vi "test.vi"() -> ()   [LabVIEW 2017]
uses:
  <vilib>/imath/engines/lvmath/Functions/Error Handling/error.ctl
  <vilib>/imath/engines/lvmath2/RunTimeEngine/Managers/WorkSpace/UID Generator.vi
  <vilib>/imath/engines/lvmath2/RunTimeEngine/NonStaticBuiltInFunctions/Manual/NIMS_NS_load.vi
  <vilib>/imath/engines/lvmath2/RunTimeEngine/NonStaticBuiltInFunctions/Manual/NIMS_NS_plot.vi
  <vilib>/imath/engines/lvmath2/RunTimeEngine/NonStaticBuiltInFunctions/NIMS_NS_hold.vi
  <vilib>/imath/engines/lvmath2/RunTimeEngine/NonStaticBuiltInFunctions/Manual/NIMS_NS_xlabel.vi
  <vilib>/imath/engines/lvmath2/RunTimeEngine/NonStaticBuiltInFunctions/Manual/NIMS_NS_ylabel.vi
  <vilib>/imath/engines/lvmath2/RunTimeEngine/NonStaticBuiltInFunctions/Manual/NIMS_NS_title.vi
  <vilib>/imath/engines/lvmath2/RunTimeEngine/NonStaticBuiltInFunctions/NIMS_NS_grid.vi
  <vilib>/imath/engines/lvmath2/RunTimeEngine/NonStaticBuiltInFunctions/Manual/NIMS_NS_legend.vi
  <vilib>/imath/engines/lvmath2/RunTimeEngine/RunTimeSymbolToken/NIMS_RunTimeSymbolToken_ResolveSymbol.vi
  <instcachedir>/0/NIMS_RunTimeSymbolToken_ResolveSymbol_AC7761ED747449B086FD7FB12AB2CB90.lvgen/NIMS_RunTimeSymbolToken_ResolveSymbol_AC7761ED747449B086FD7FB12AB2CB90_003.vi
  <vilib>/imath/engines/lvmath2/RunTimeEngine/Managers/SymbolTable/Write Variable.vi
  <vilib>/imath/engines/lvmath2/RunTimeEngine/Managers/SymbolTable/Read Variable.vi
  <vilib>/imath/engines/lvmath2/RunTimeEngine/VariableToken/Read/NIMS_Get Elements - _($,_) - nonstatic.vi
  <vilib>/imath/engines/lvmath2/RunTimeEngine/RunTimeSymbolToken/NIMS_RunTimeSymbolToken_UserFunctionInvoke.vi
  <vilib>/imathl/engines/lvmath/Functions/Error Handling/Create Error.vi
  <vilib>/imath/engines/lvmath2/RunTimeEngine/ArithmeticOperatorToken/NIMS_NS_ArithmeticOperator_times.vi
  <vilib>/imath/engines/lvmath/Functions/Error Handling/MergeErrorsWrapper.vi
  <instcachedir>/0/NIMS_RunTimeSymbolToken_ResolveSymbol_AC7761ED747449B086FD7FB12AB2CB90.lvgen/NIMS_RunTimeSymbolToken_ResolveSymbol_AC7761ED747449B086FD7FB12AB2CB90_002.vi
  <instcachedir>/0/NIMS_RunTimeSymbolToken_ResolveSymbol_AC7761ED747449B086FD7FB12AB2CB90.lvgen/NIMS_RunTimeSymbolToken_ResolveSymbol_AC7761ED747449B086FD7FB12AB2CB90_000.vi
  <vilib>/imath/engines/lvmath2/RunTimeEngine/CommandStatement/NIMS_CommandStatement_MaskErr.vi
  <vilib>/imath/engines/lvmath2/RunTimeEngine/NodeEndStatement/MC_NodeEndStatement_Dispose.vi
  <vilib>/imath/engines/lvmath2/RunTimeEngine/ErrorHandling/NIMS_Finalize Error.vi
  <vilib>/imath/engines/lvmath2/RunTimeEngine/ArithmeticOperatorToken/NIMS_NS_ArithmeticOperator_plus.vi
  <vilib>/imath/engines/lvmath2/RunTimeEngine/ArithmeticOperatorToken/NIMS_NS_ArithmeticOperator_minus.vi
  <vilib>/imath/engines/lvmath2/RunTimeEngine/Managers/SymbolTable/NIMS_WorkSpace.lvlib
panel:
  in  "还原按钮":bool
  in  "电机工作频率":dbl
  in  "预紧力":dbl
  in  "转子光电总阻尼":dbl
  in  "轴向阻尼系数":dbl
  in  "转子等效半径":dbl
  in  "输入完成":bool
  in  "摩擦材料等效刚度":dbl
  in  "定转子间动摩擦系数":dbl
  in  "行波波数":dbl
  out "loading":T1 caption="Loading..." scale=0.0..100.0
  in  "摩擦转矩-转速":bool
  in  "启动特性":bool
  in  "完成":bool
  in  "完成":bool
  in  "完成":bool
  in  "矩角特性":bool
  in  "?":bool
  in  "?":bool
  in  "?":bool
  in  "定子形波振幅3":dbl
  in  "定子形波振幅2":dbl
  in  "定子形波振幅":dbl
  in  "启动特性":bool
  in  "完成":bool
  in  "?":bool
  in  "负载转矩4":dbl
  in  "完成":bool
  in  "完成":bool
  in  "完成":bool
  in  "矩角特性":bool
  in  "净输出转矩-转速关系":bool
  in  "?":bool
  in  "?":bool
  in  "?":bool
  in  "负载转矩3":dbl
  in  "负载转矩2":dbl
  in  "负载转矩1":dbl
  in  "完成":bool
  in  "完成":bool
  in  "完成":bool
  in  "启动特性":bool
  in  "矩角特性":bool
  in  "?":bool
  in  "?":bool
  in  "?":bool
  in  "转动惯量":dbl
  in  "转动惯量":dbl
  in  "转动惯量":dbl
  # "瞬态特性测试模块"
  # "负载转矩"
  # "电机参数"
  # "负载转动惯量"
  # "定子行波振幅"
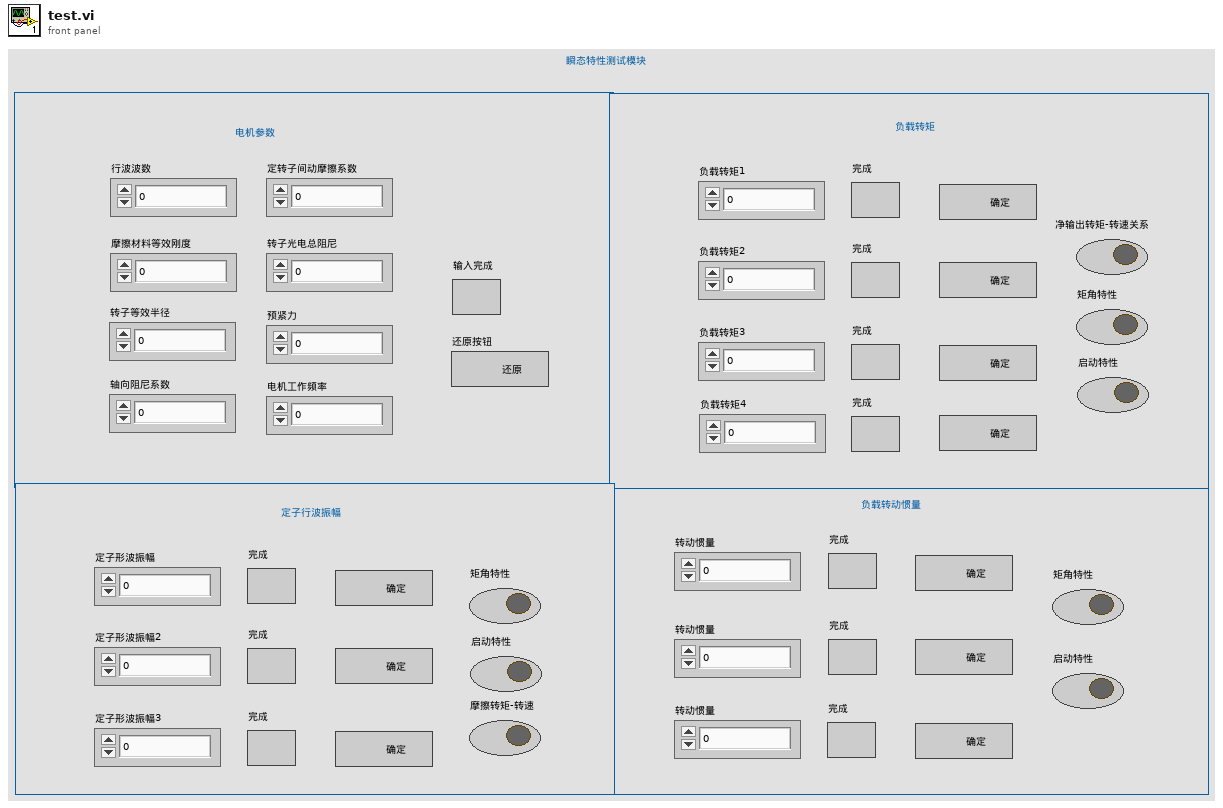
[diagram p1: front panel]
types:
  T1 = typedef "控件 1.ctl" = u8
  T2 = enum16{"open", "replace", "create", "open or create", "replace or create", "replace or create with confirmation"}
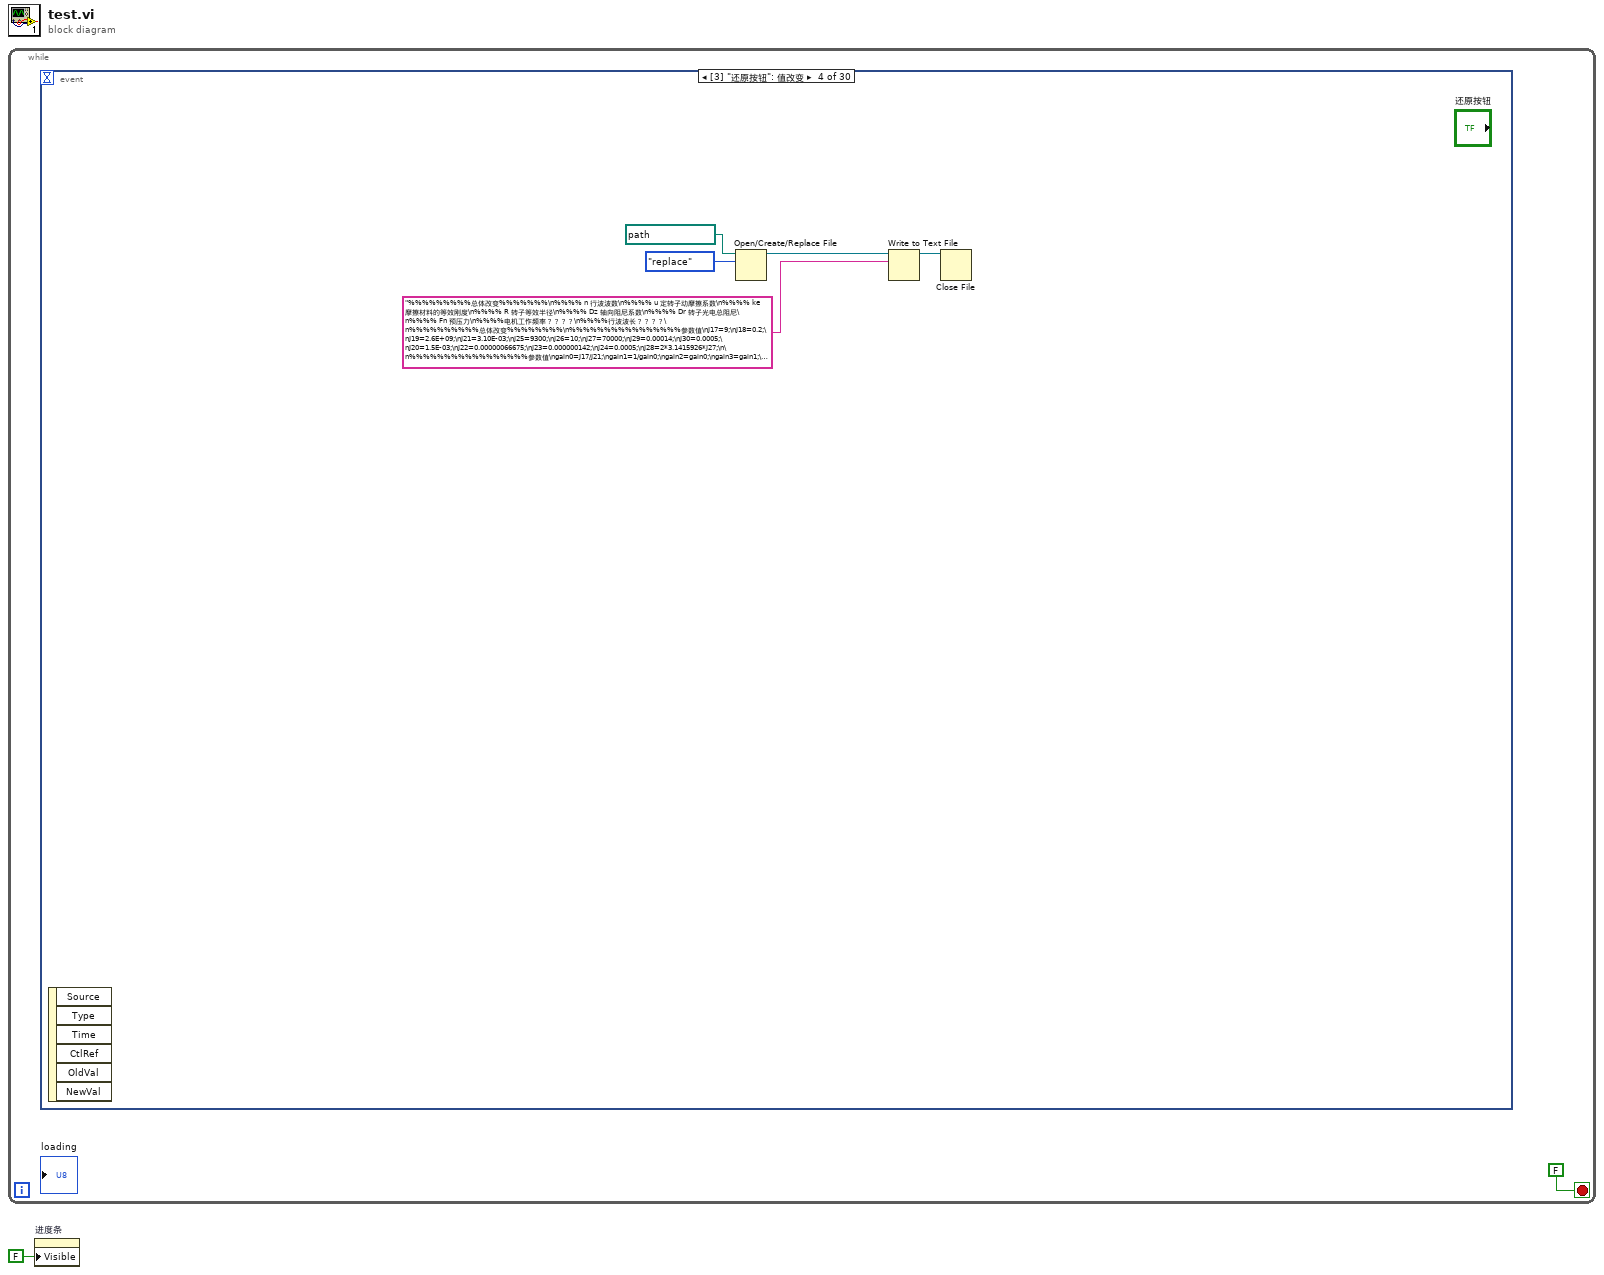
[diagram p0: block diagram]
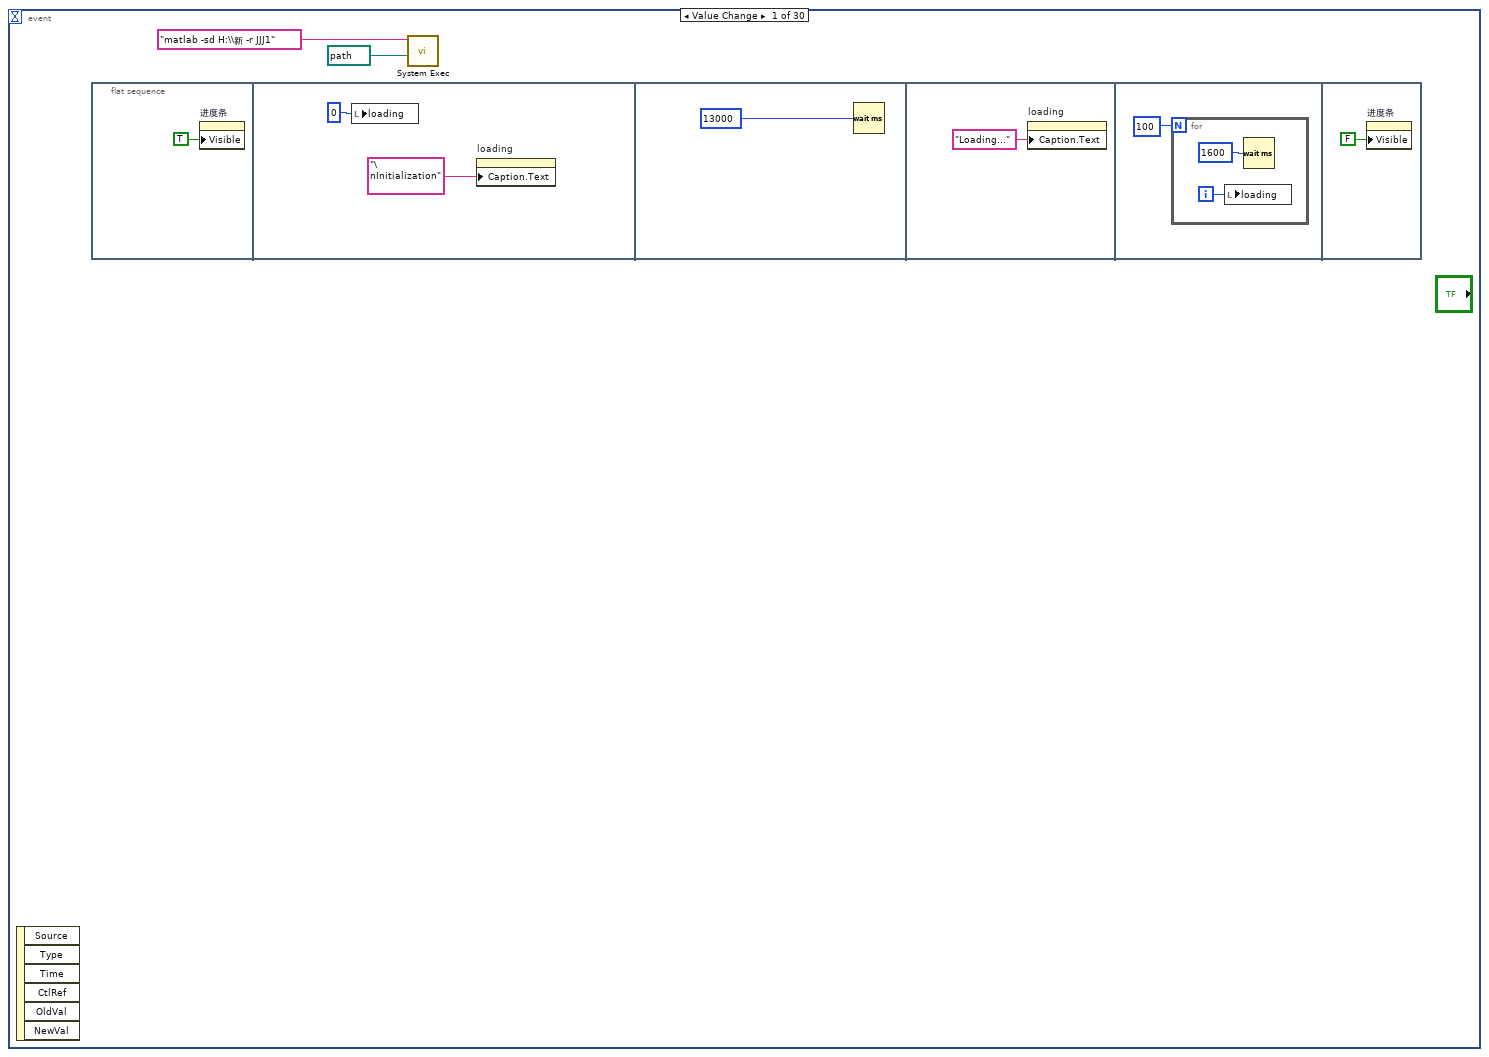
[diagram p2: hidden frame]
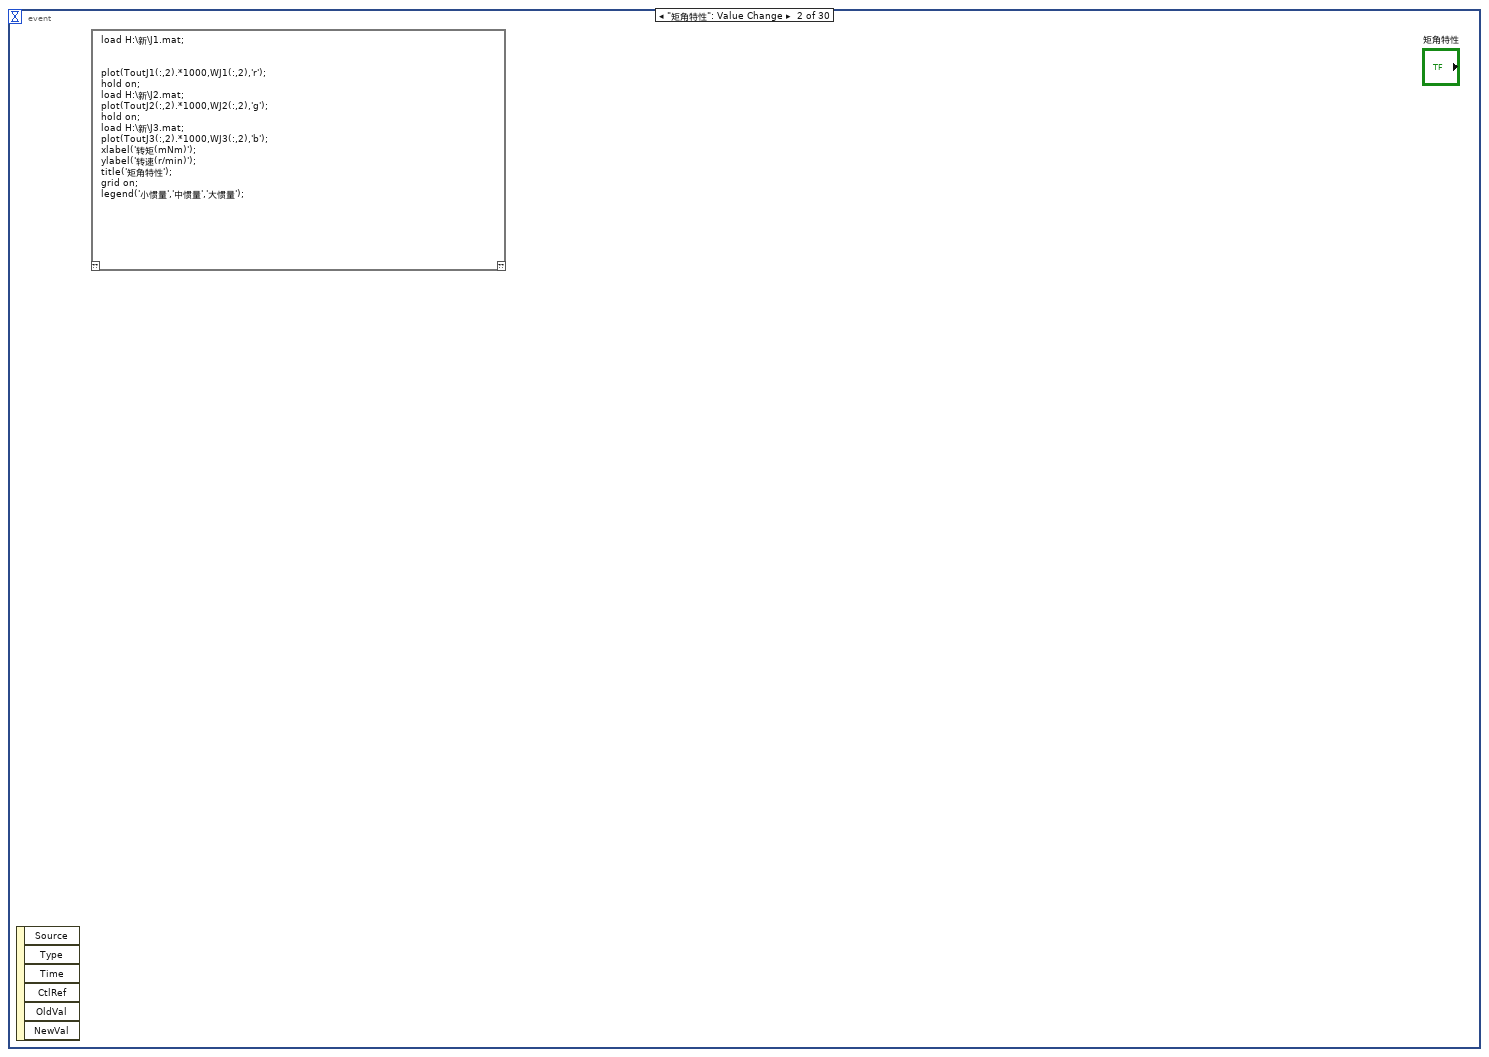
[diagram p3: hidden frame]
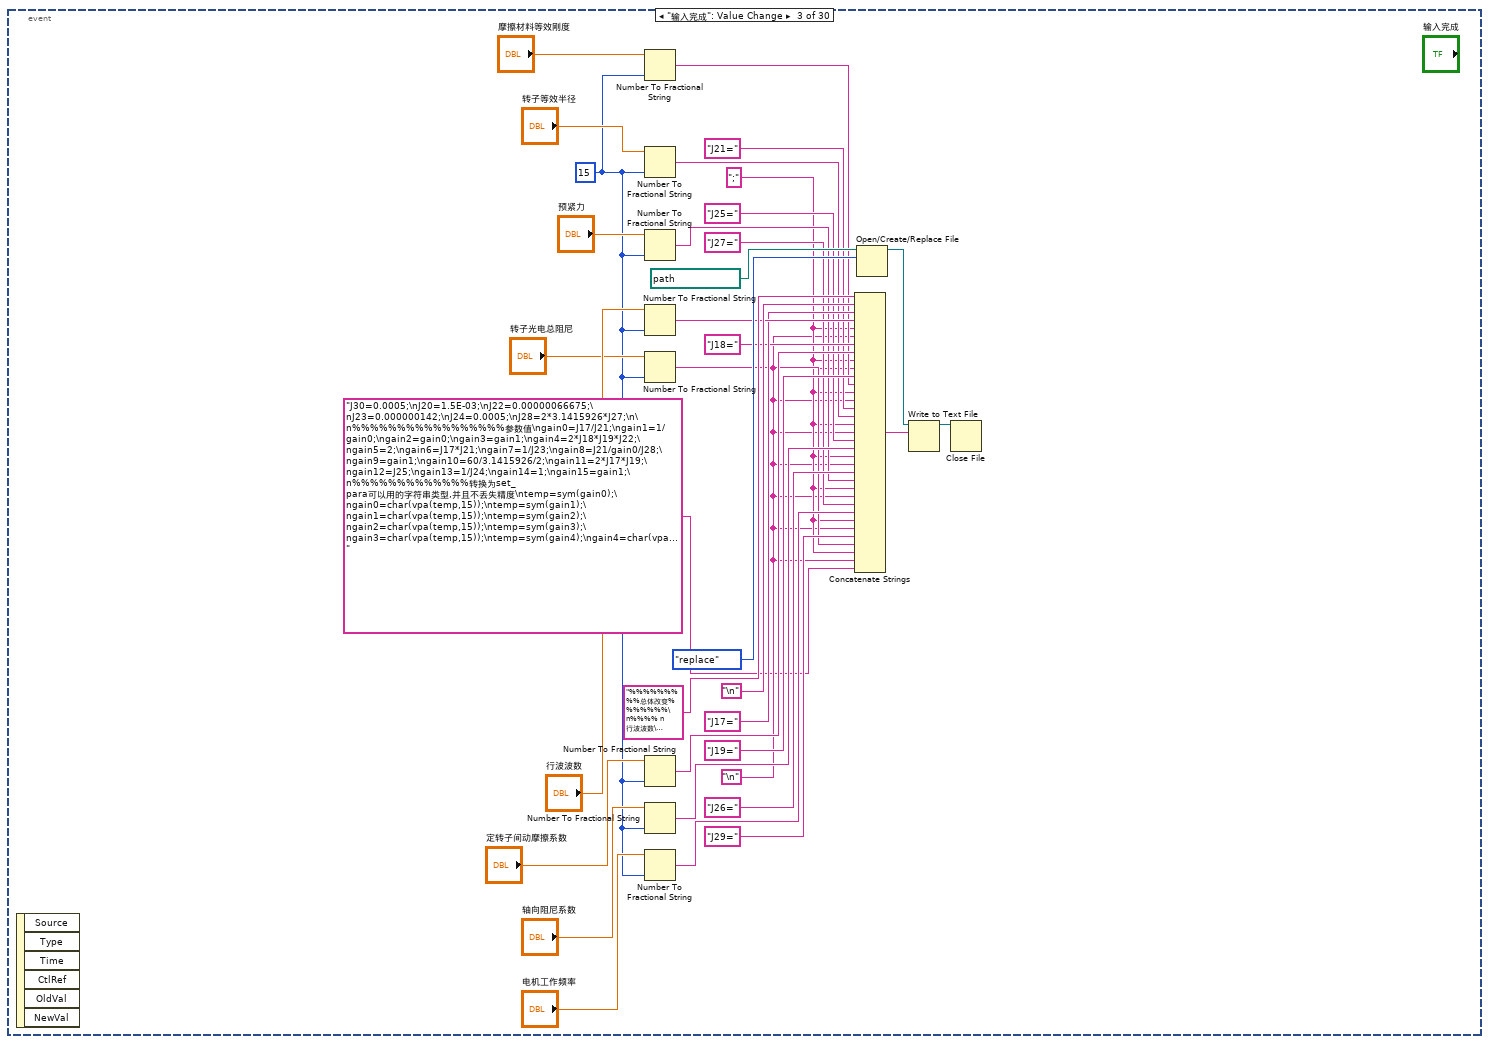
[diagram p4: hidden frame]
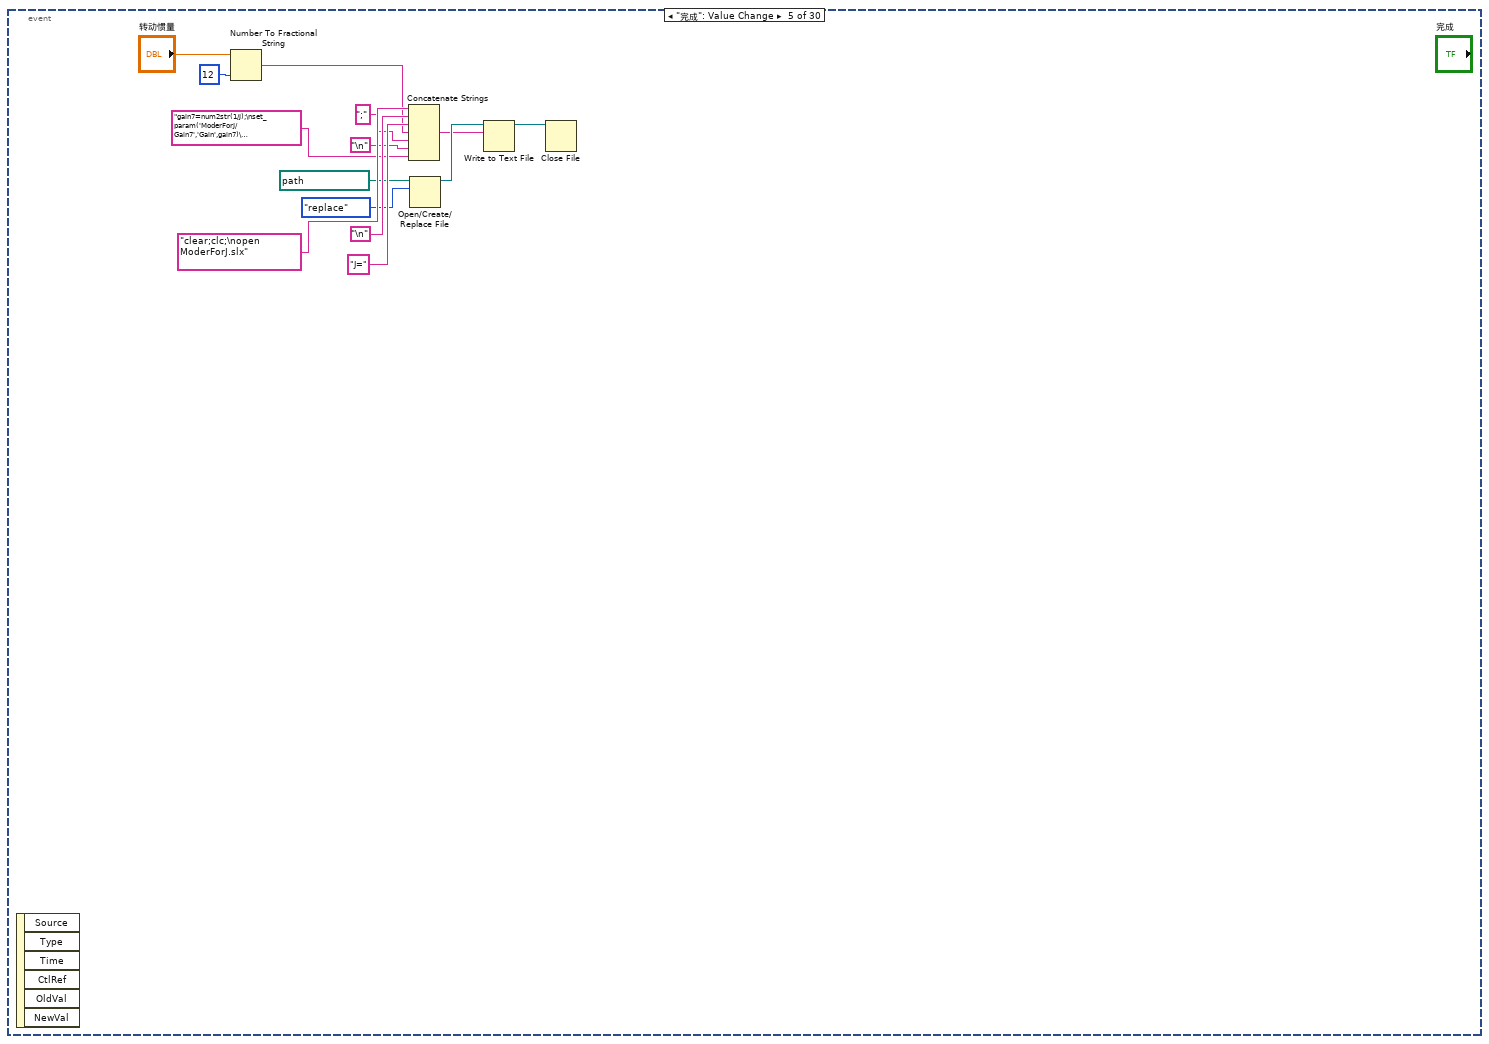
[diagram p5: hidden frame]
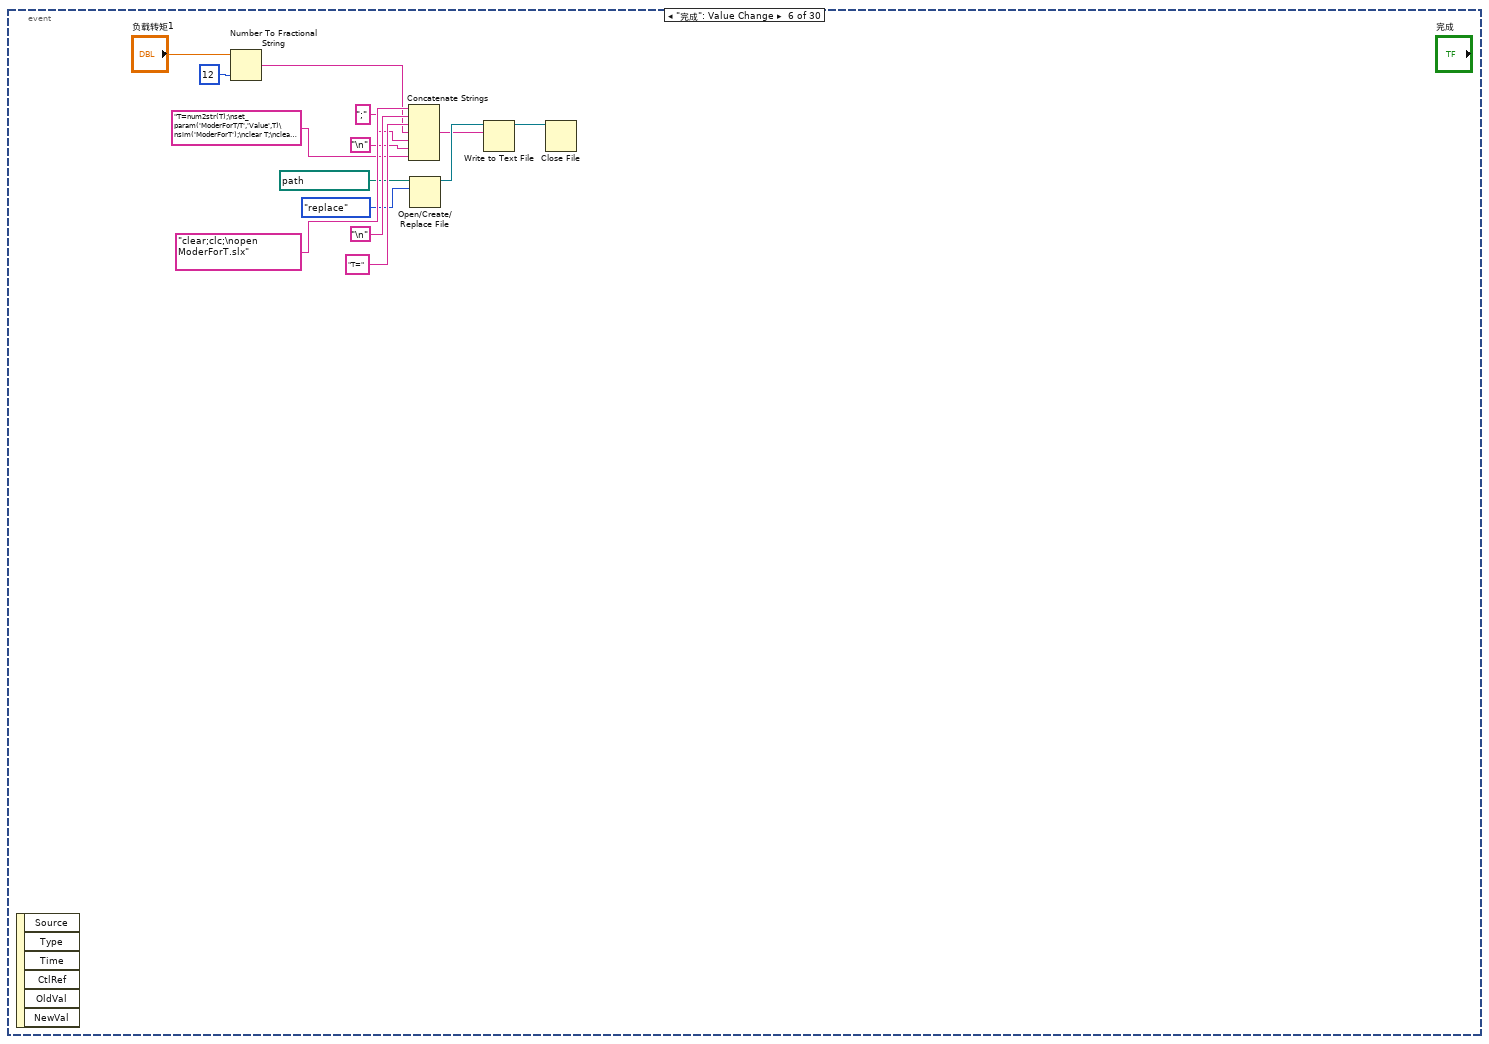
[diagram p6: hidden frame]
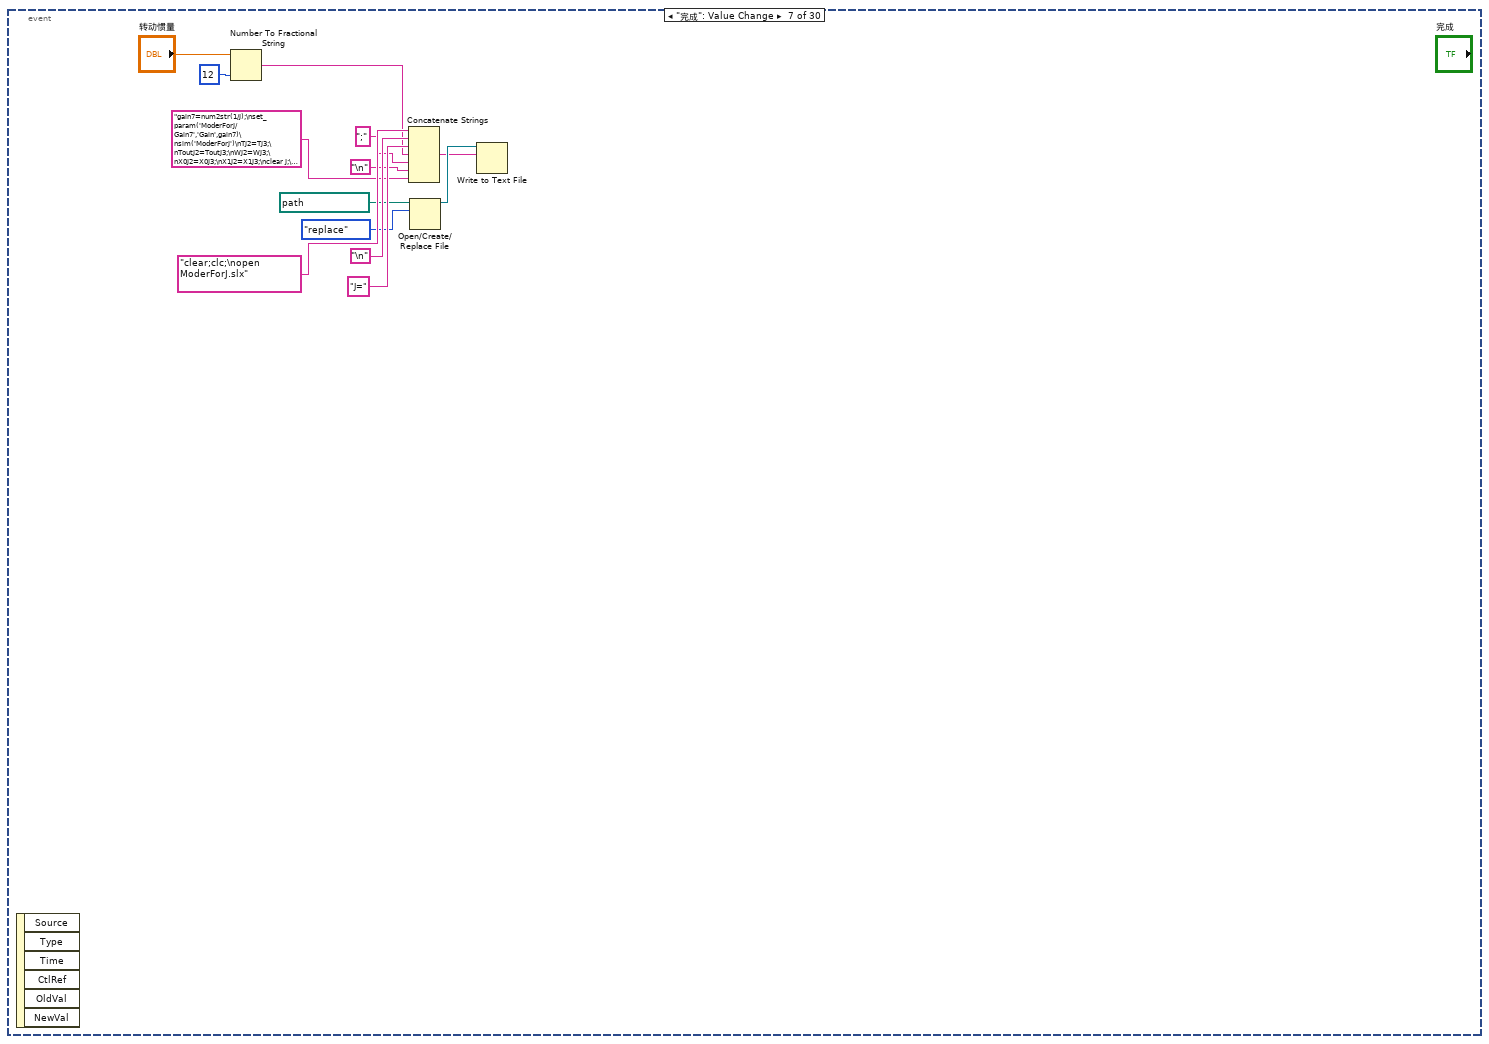
[diagram p7: hidden frame]
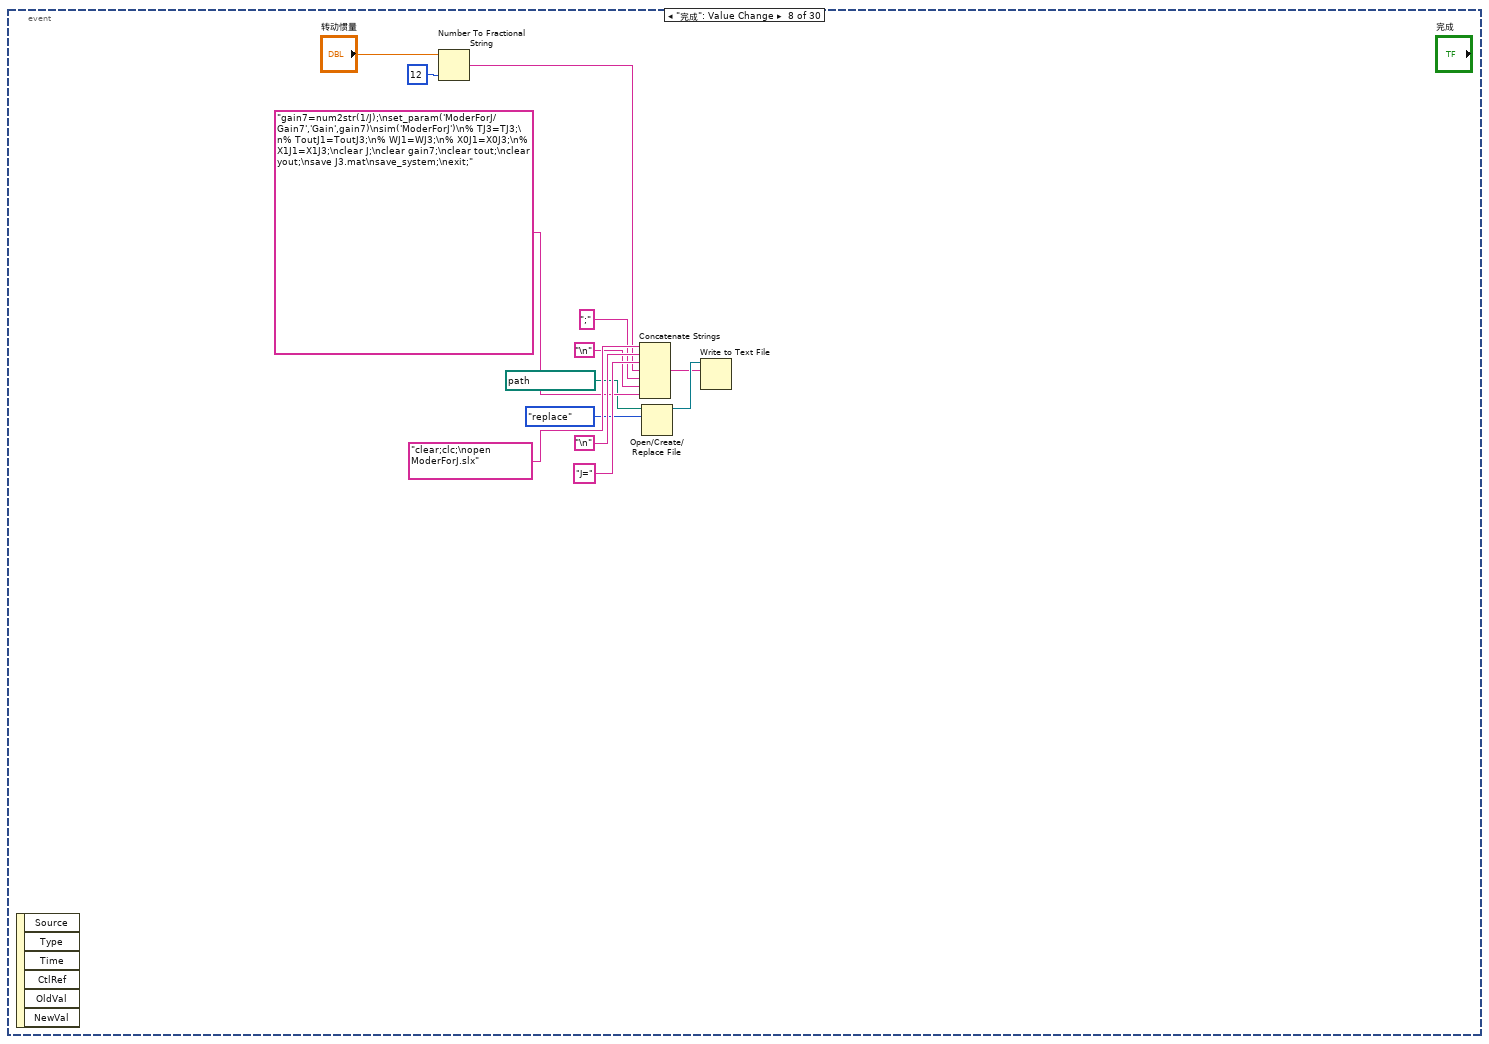
[diagram p8: hidden frame]
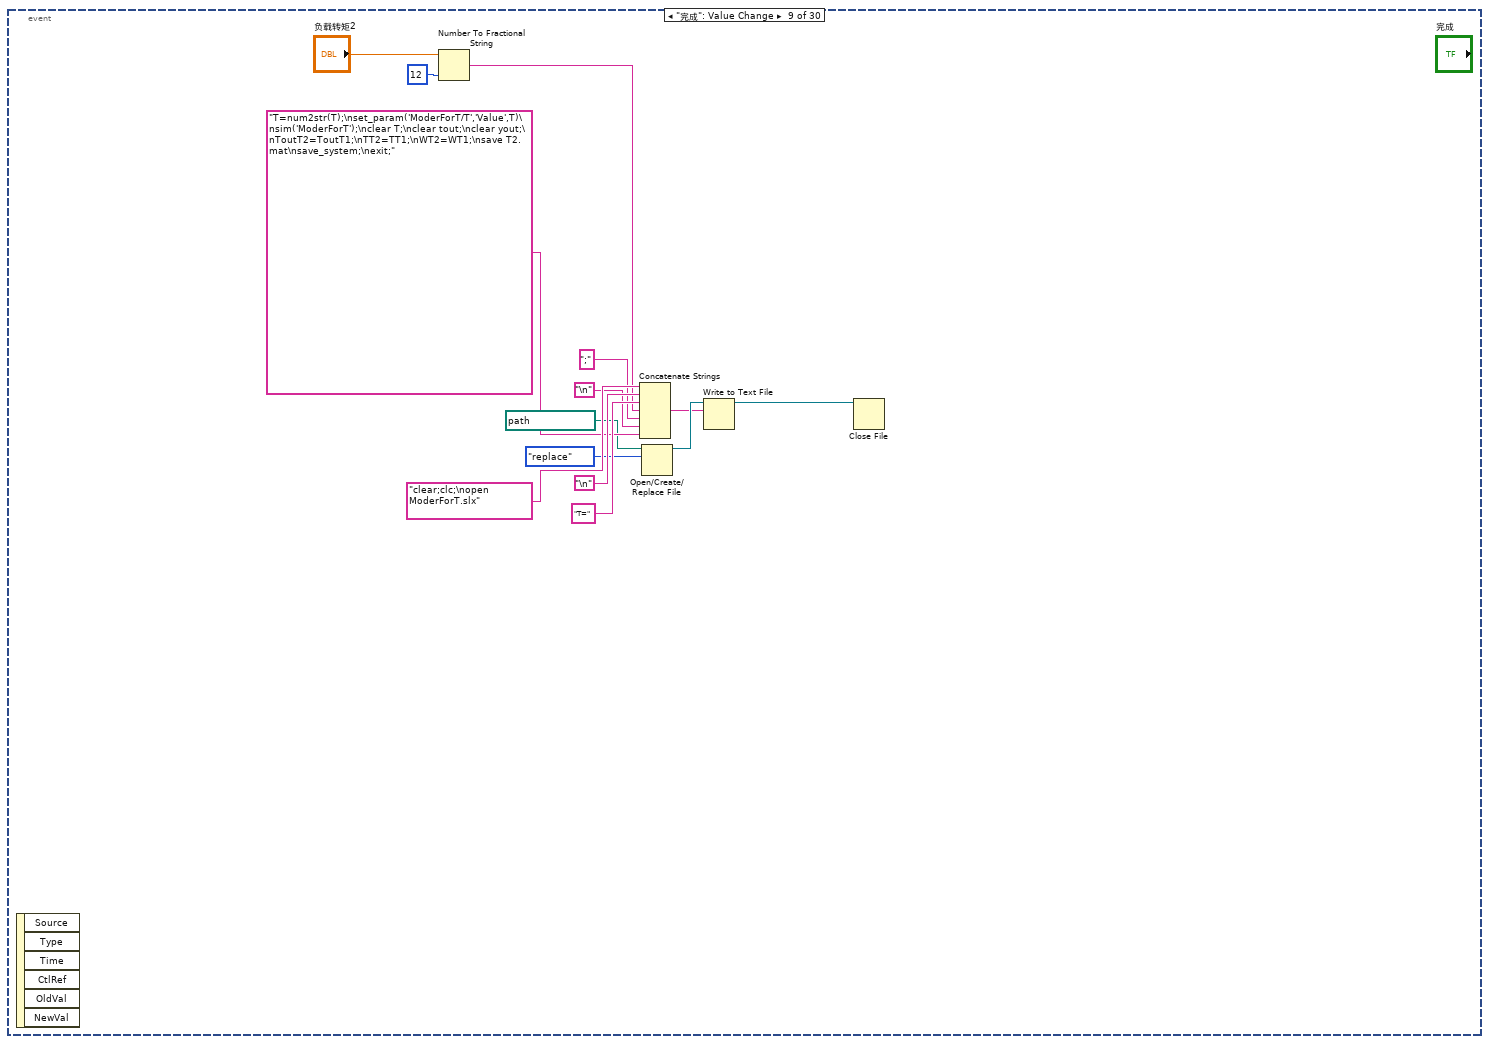
[diagram p9: hidden frame]
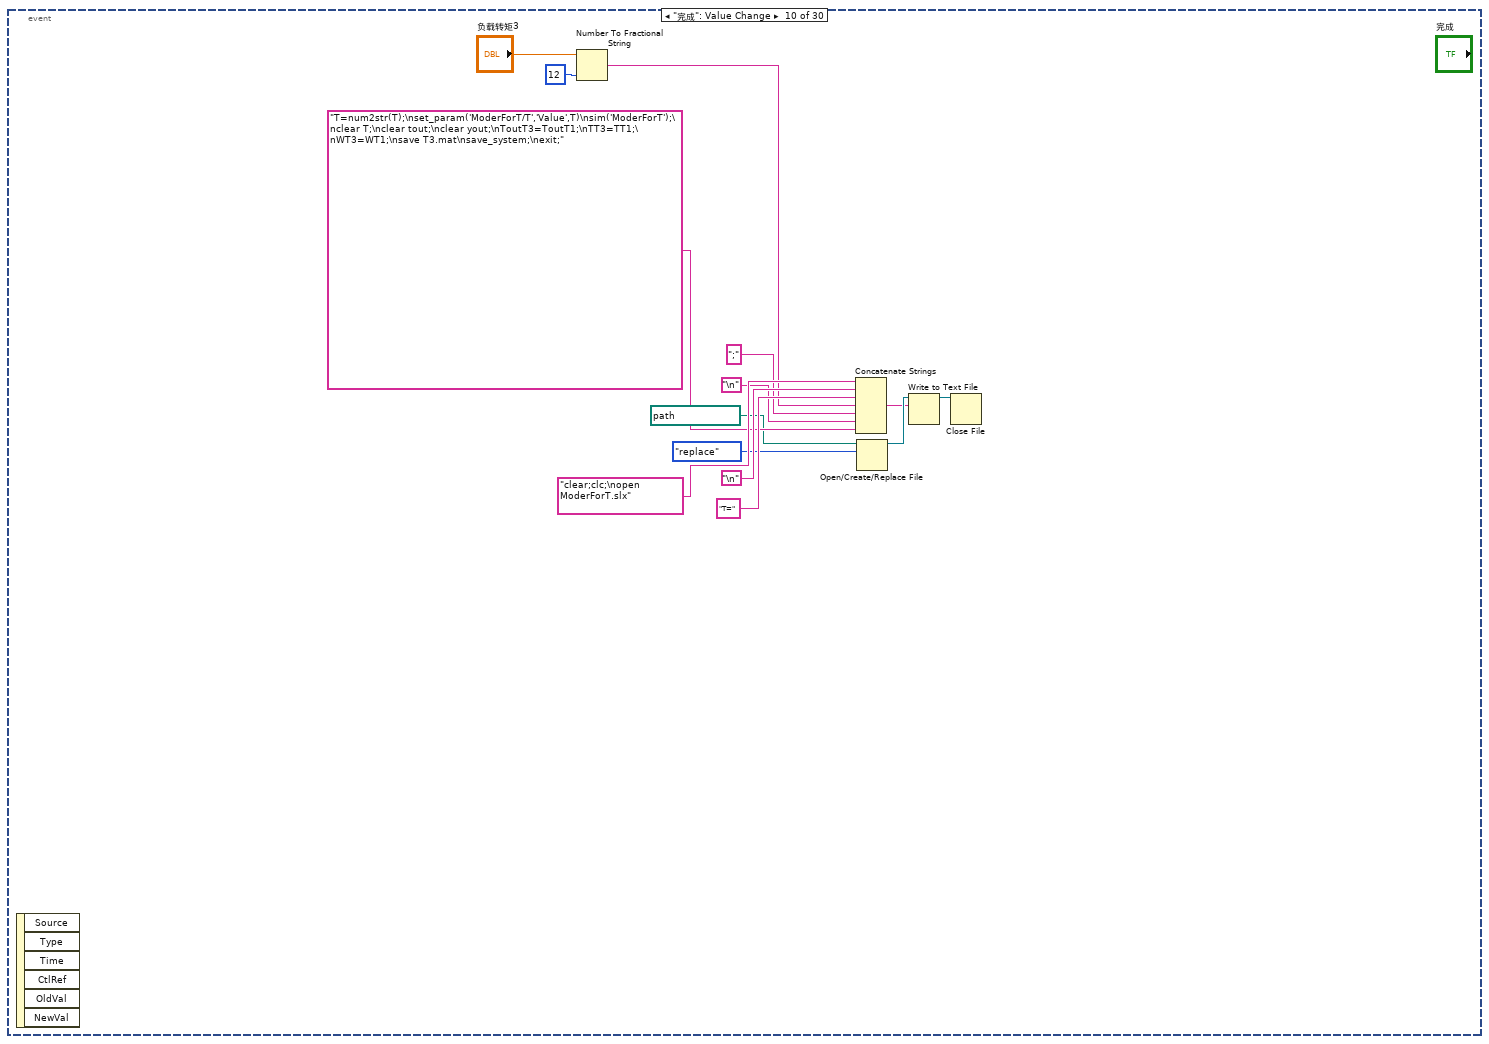
[diagram p10: hidden frame]
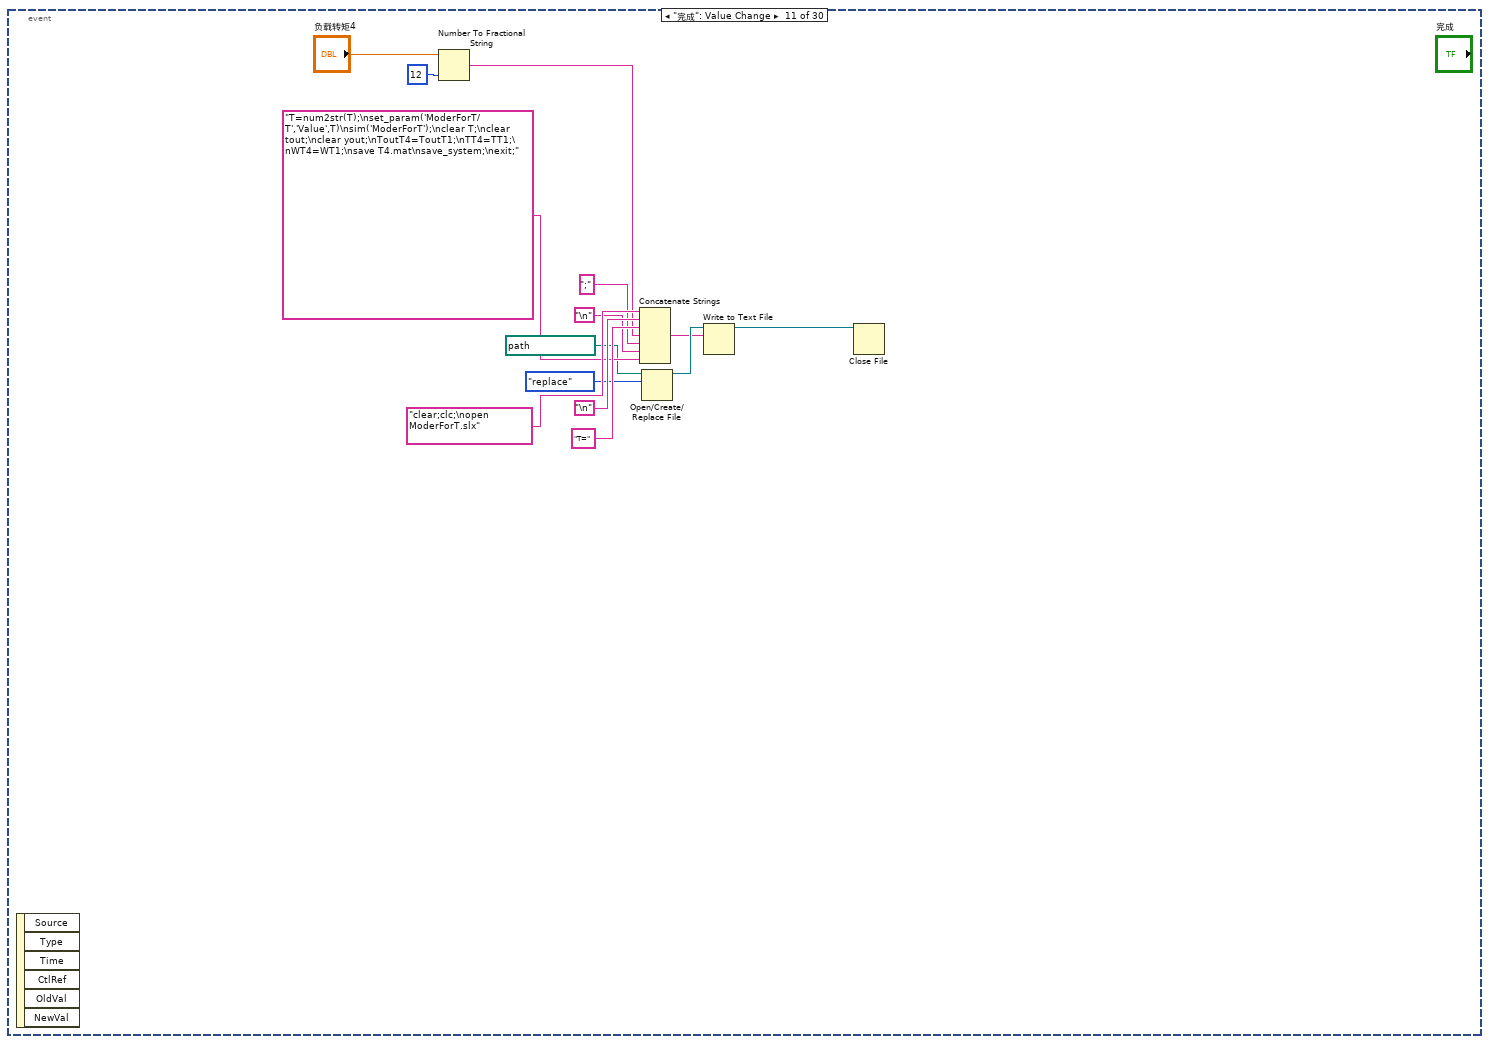
[diagram p11: hidden frame]
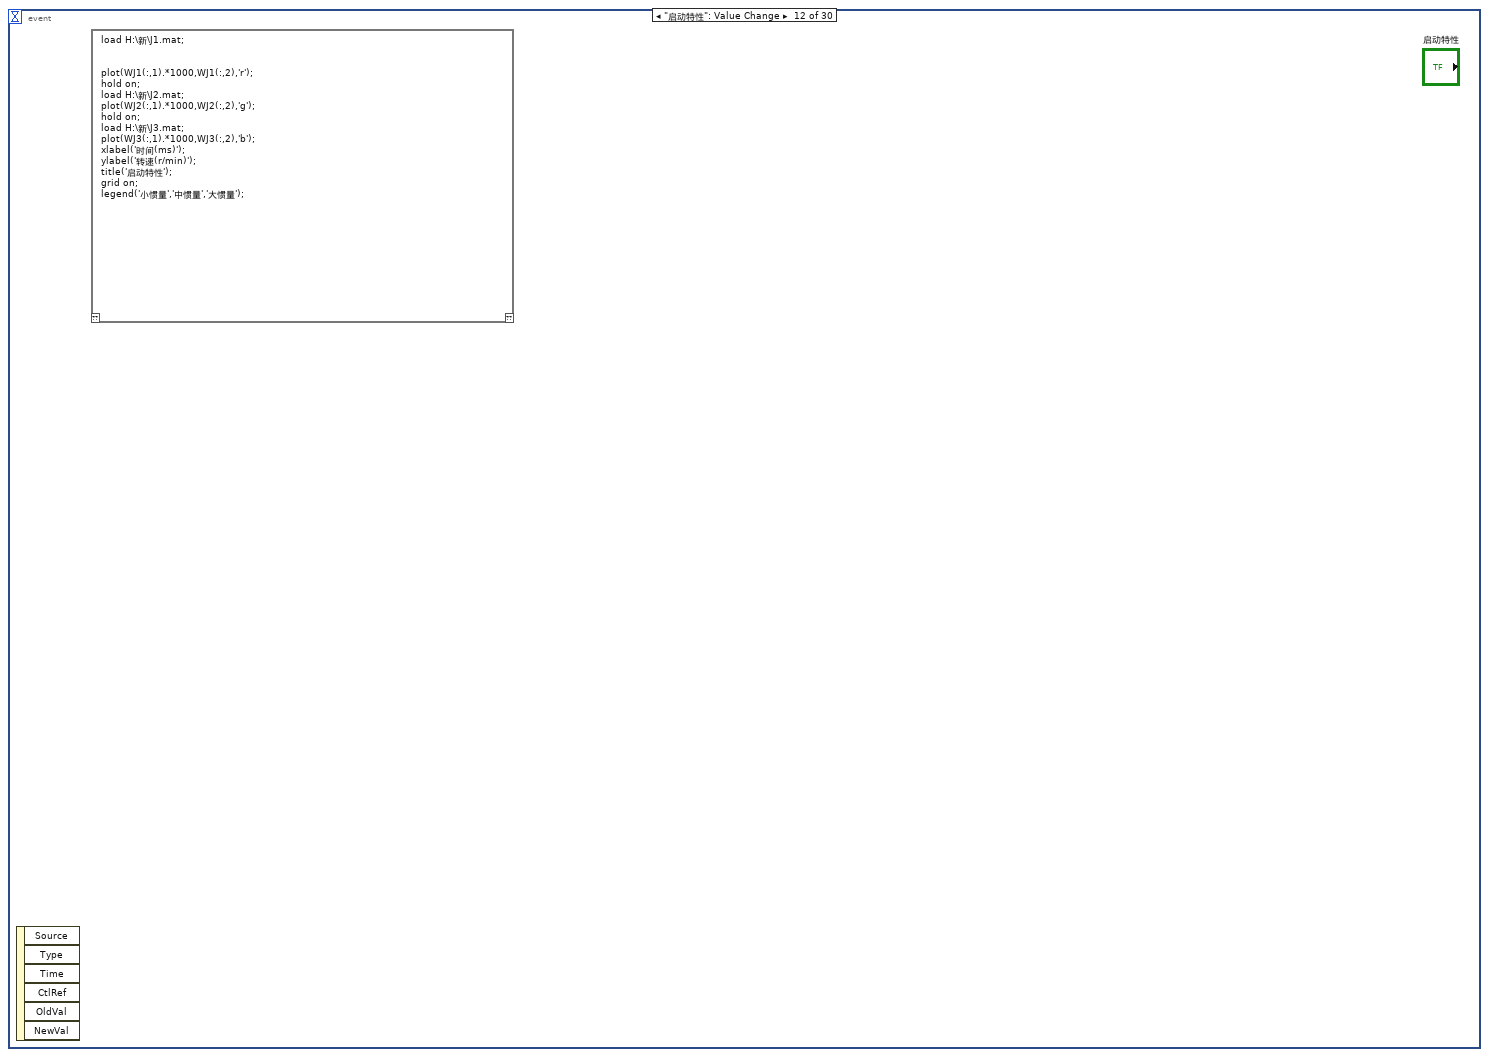
[diagram p12: hidden frame]
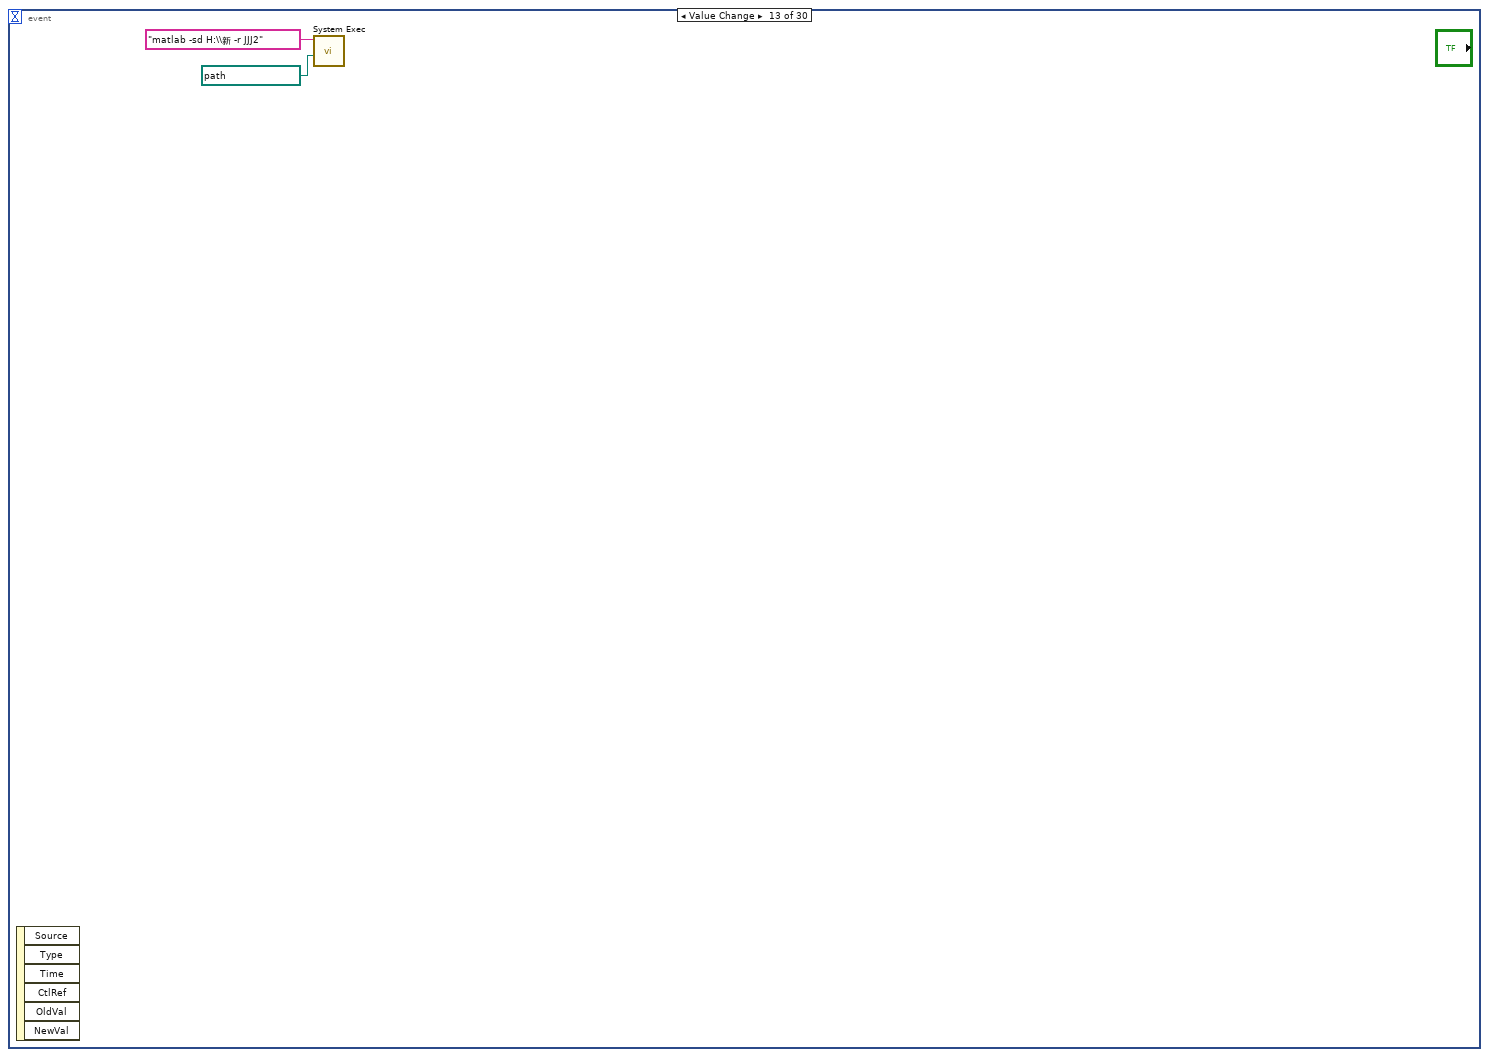
[diagram p13: hidden frame]
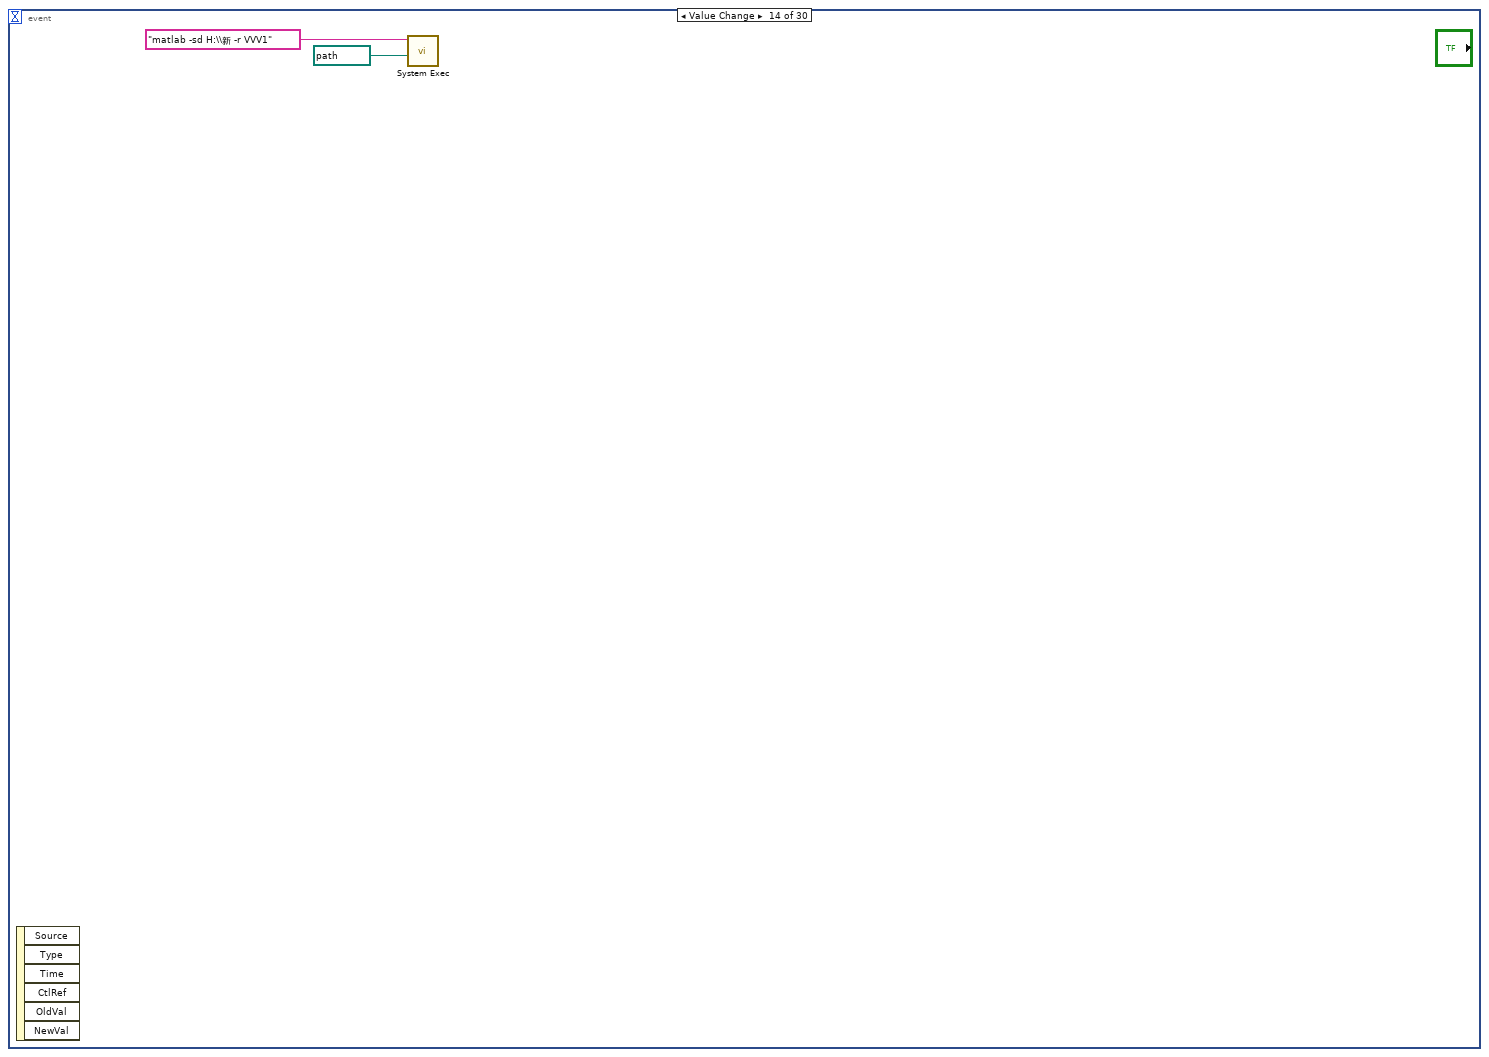
[diagram p14: hidden frame]
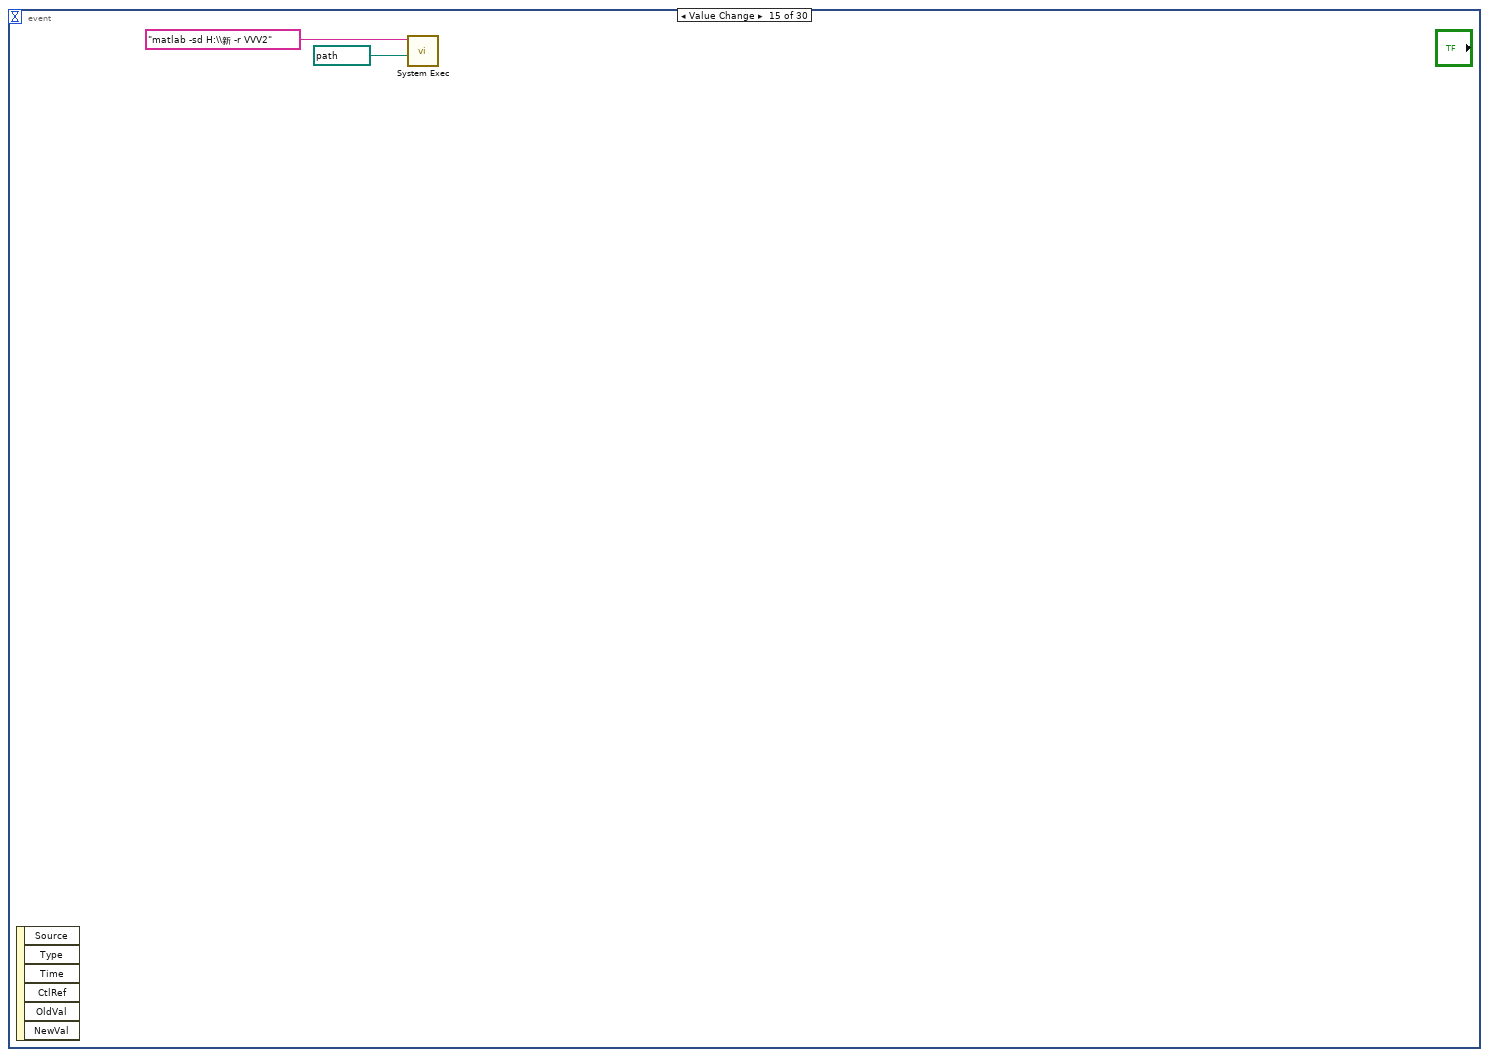
[diagram p15: hidden frame]
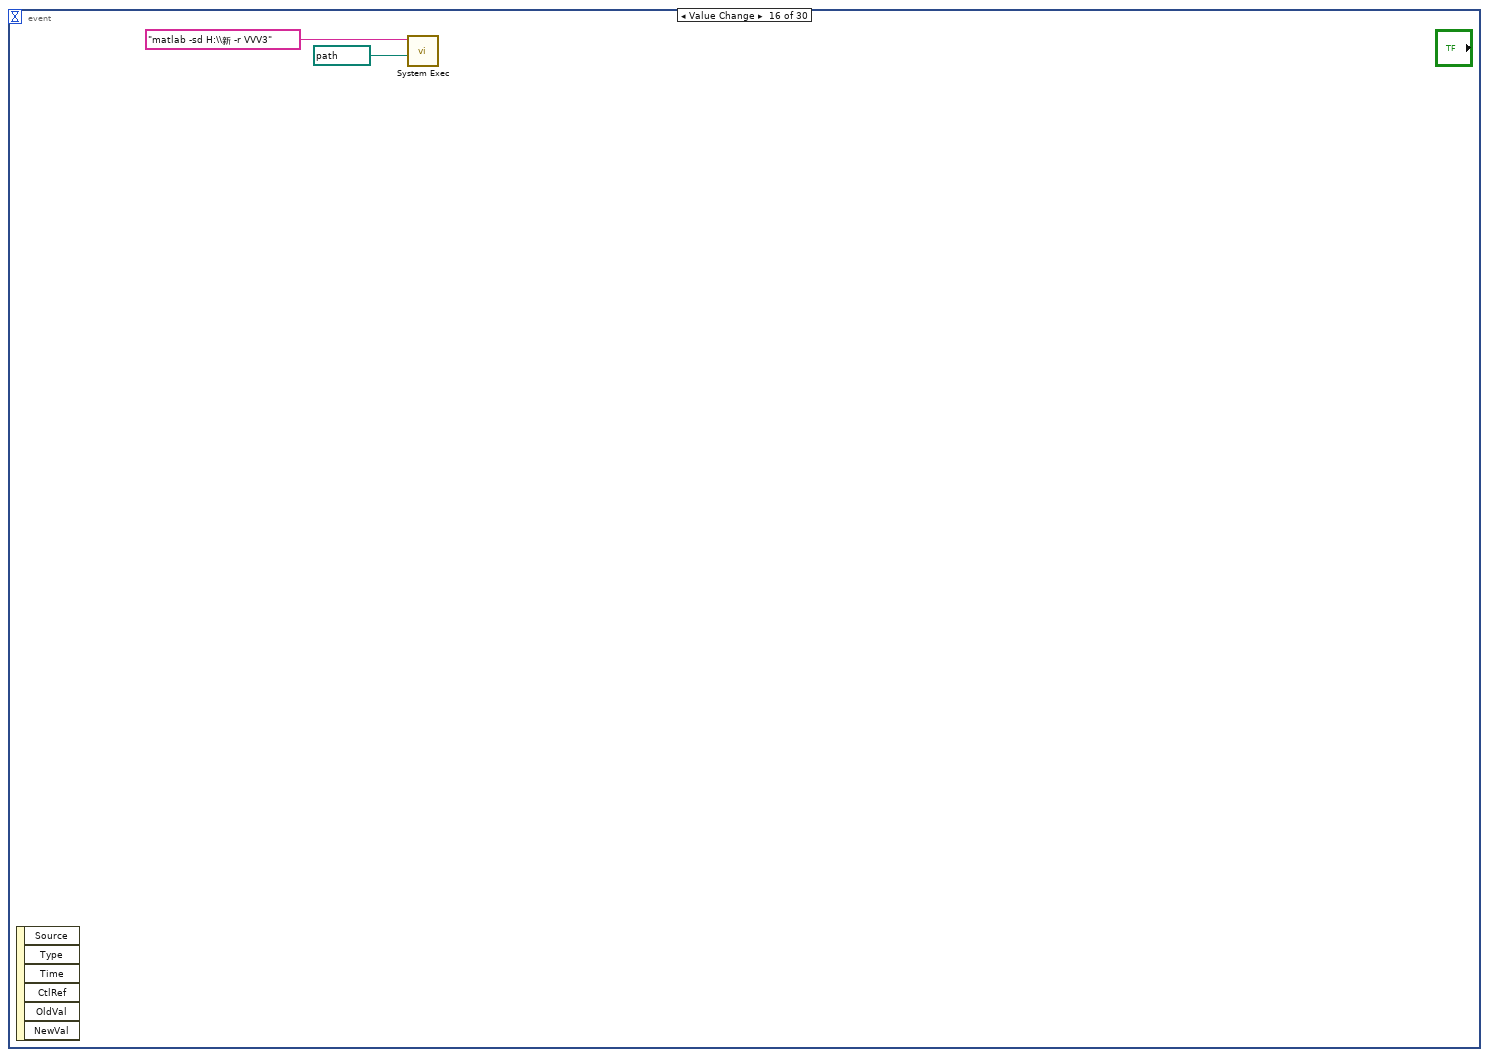
[diagram p16: hidden frame]
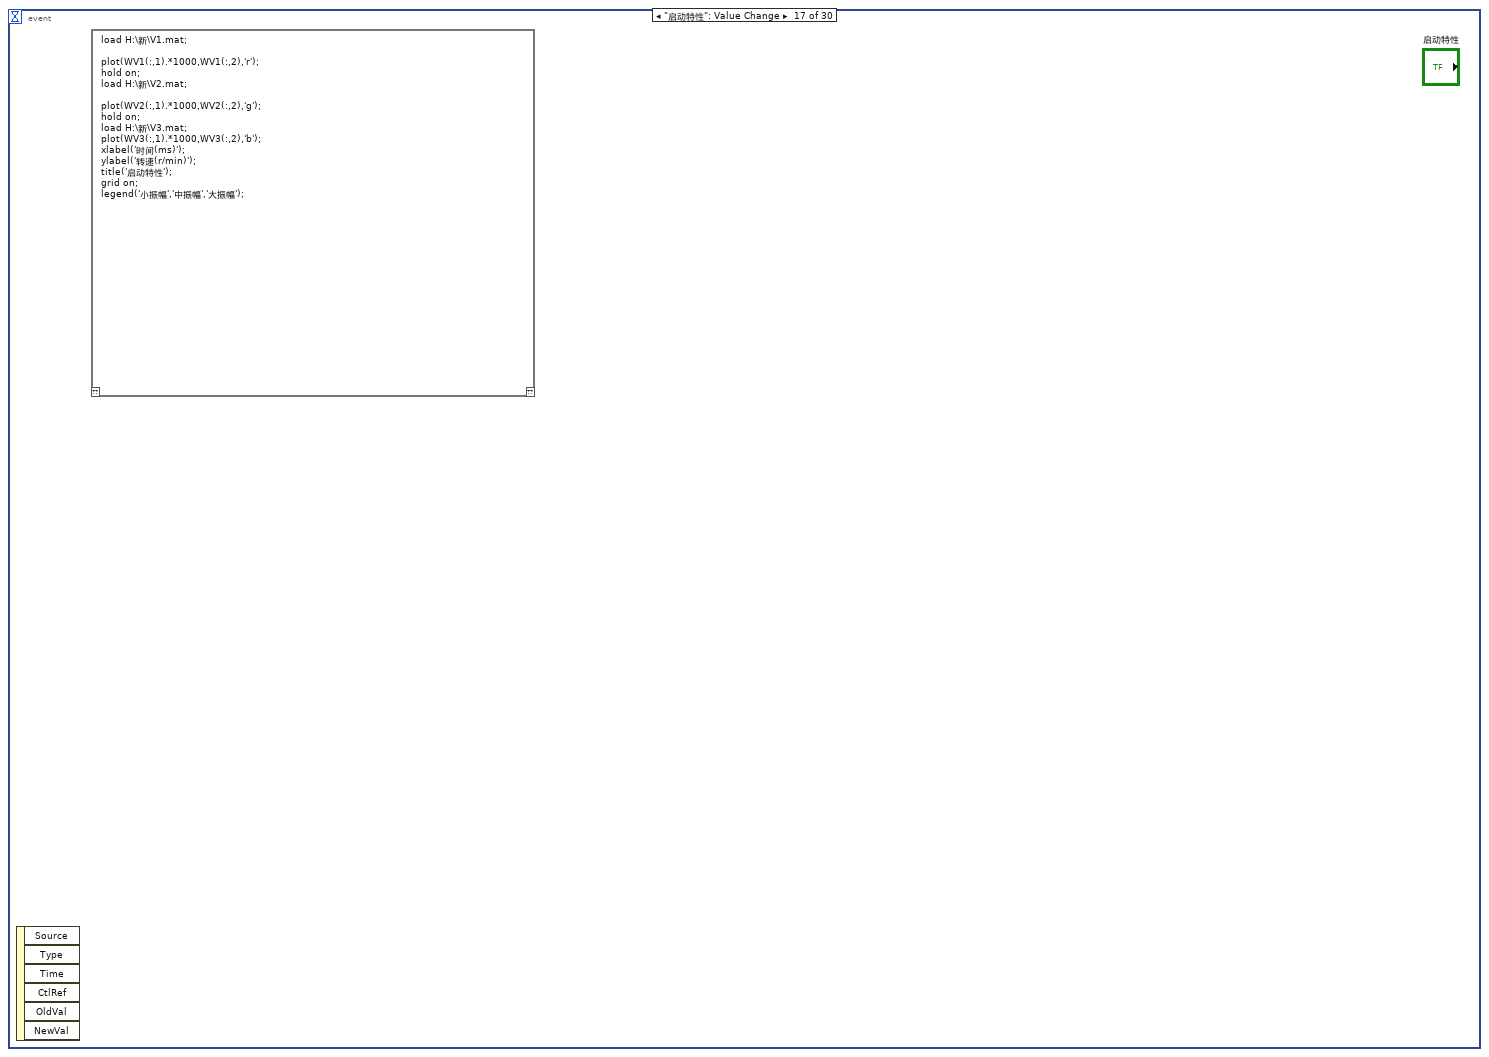
[diagram p17: hidden frame]
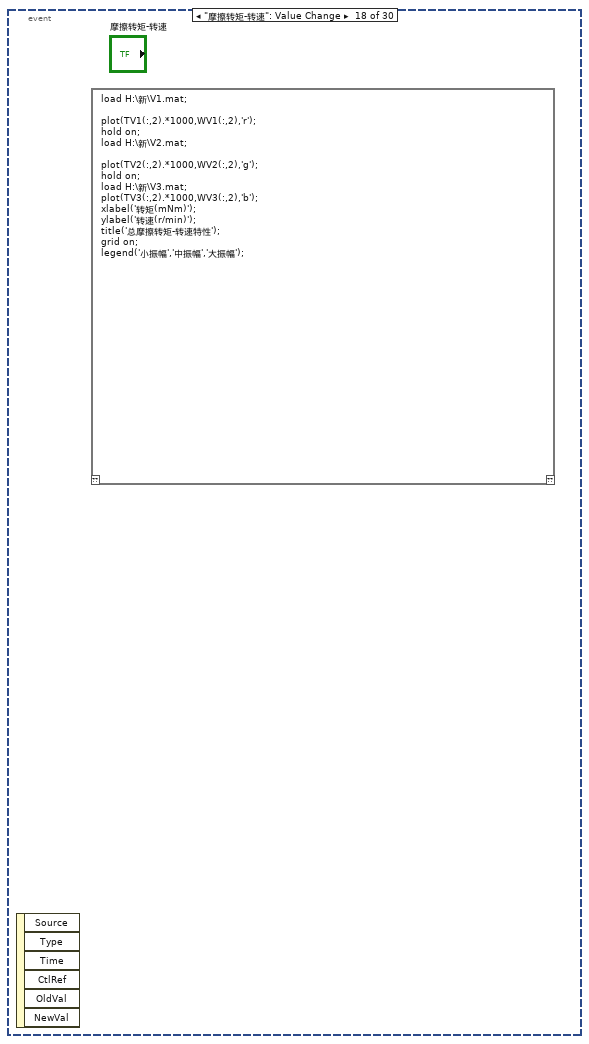
[diagram p18: hidden frame]
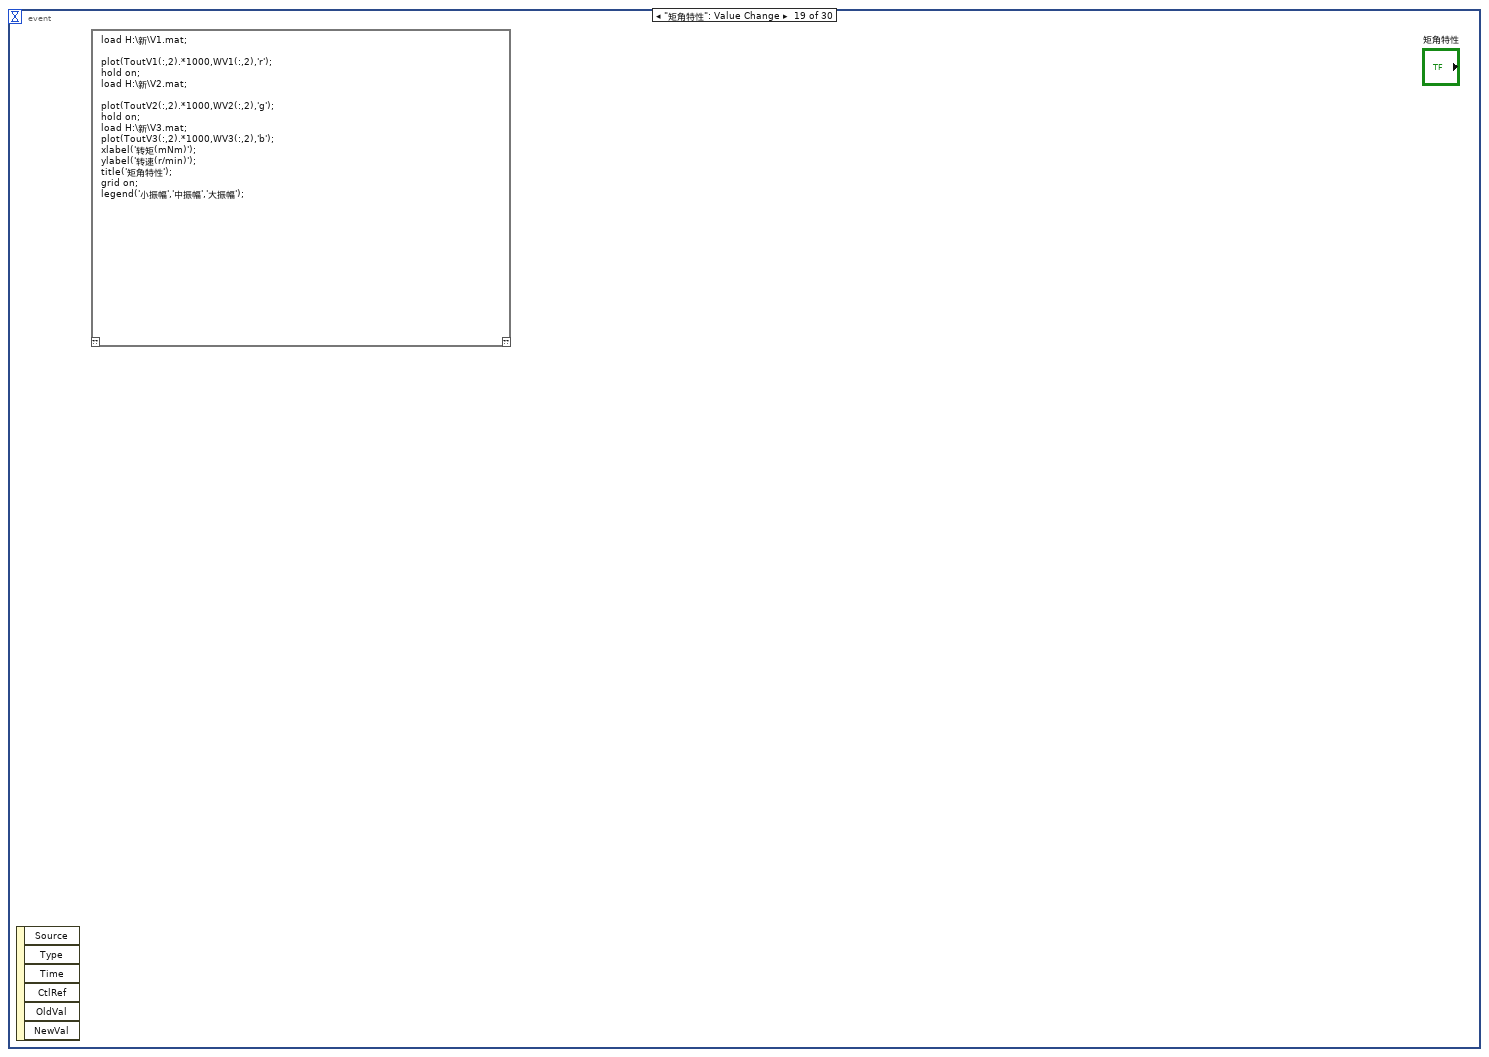
[diagram p19: hidden frame]
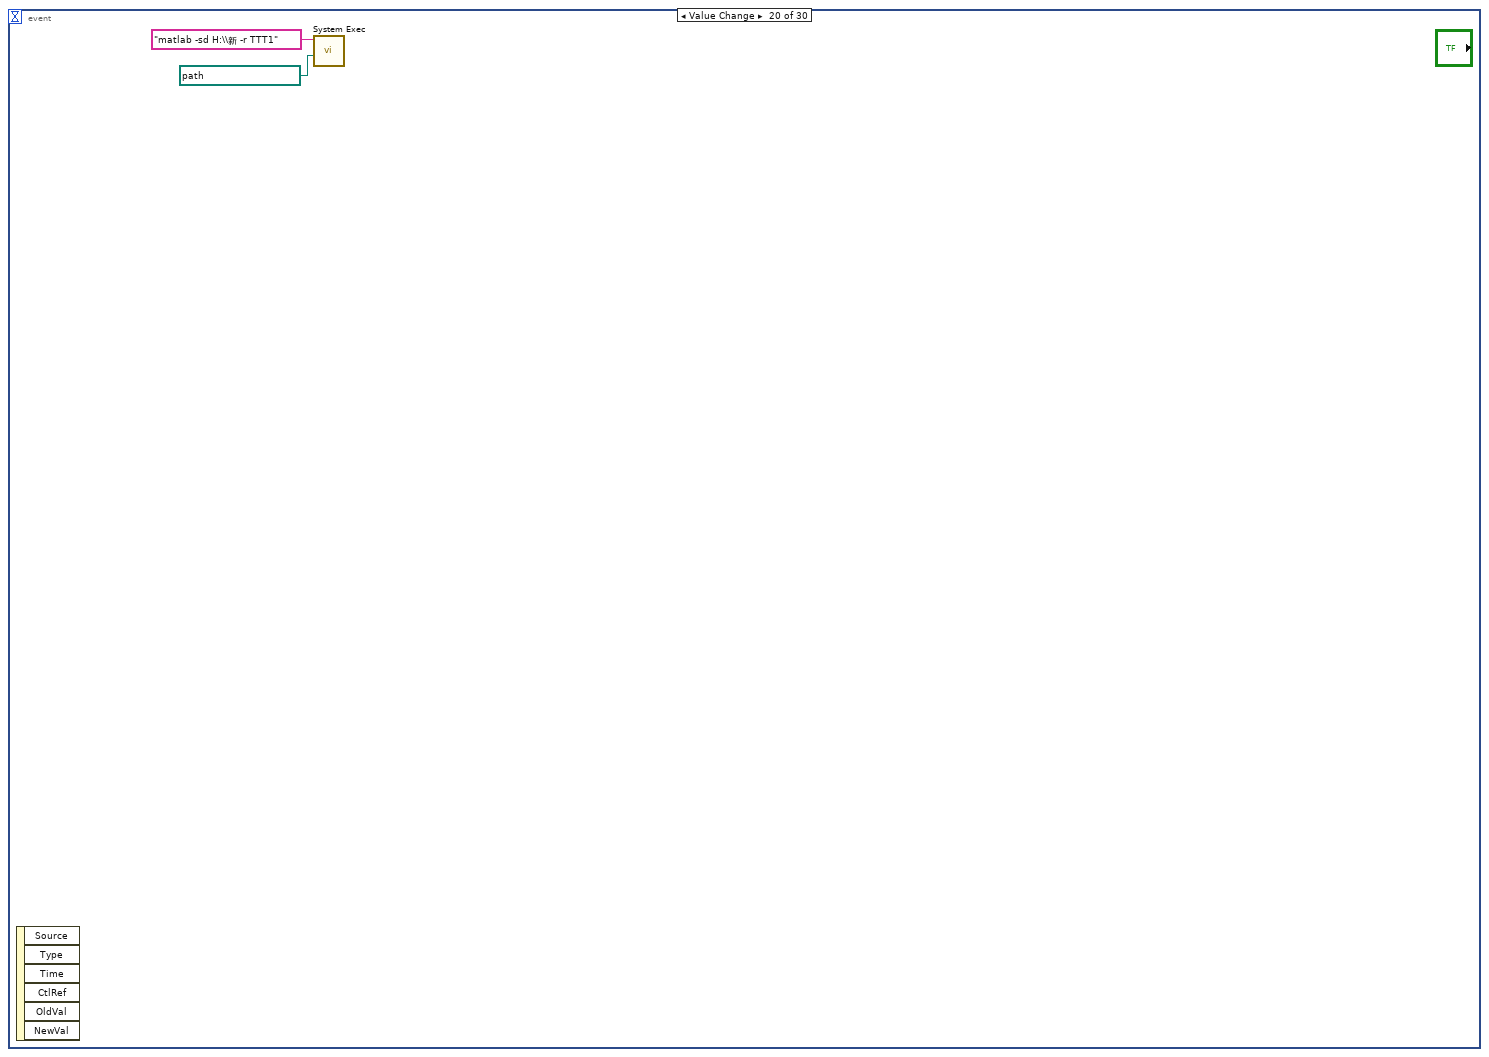
[diagram p20: hidden frame]
diagram:
  n1 = while {
    stop <- FALSE stop-if-true
    n2 = event shown="[3] \"还原按钮\": 值改变" {
      selector: _ -> [_ _ _ _ _ _ _ _ _ _ _ _ _ _ _ _ _ _ _ _ _ _ _ _ _ _ _ _ _ _]
      dyn-events: _ -> [_ _ _ _ _ _ _ _ _ _ _ _ _ _ _ _ _ _ _ _ _ _ _ _ _ _ _ _ _ _]
      timeout: _ -> [_ _ _ _ _ _ _ _ _ _ _ _ _ _ _ _ _ _ _ _ _ _ _ _ _ _ _ _ _ _]
      event Value Change {
        n3 = event-data() -> ()  [unwired: 1 in, 6 out]
        n4 = flat-sequence {
          frame #0 {
            n5 = property on="进度条" class="Slide (严格)"("Visible"=TRUE ("可见")) -> ()  [unwired: 2 in, 2 out]
          }
          frame #1 {
            n6 = local write "loading"(T1 0 ("进度条")) -> ()
            n7 = property on="loading" class="Slide (严格)"("Caption.Text"="\nInitialization" ("标题.文本")) -> ()  [unwired: 2 in, 2 out]
          }
          frame #2 {
            n8 = Wait (ms)(milliseconds to wait=u32 13000 ("等待时间（毫秒）")) -> ()  [unwired: 1 out]
          }
          frame #3 {
            n9 = property on="loading" class="Slide (严格)"("Caption.Text"="Loading..." ("标题.文本")) -> ()  [unwired: 2 in, 2 out]
          }
          frame #4 {
            n10 = for {
              N: 100 -> [_]
              i -> [w11]
              n11 = local write "loading"(w11) -> ()
              n12 = Wait (ms)(milliseconds to wait=u32 1600 ("等待时间（毫秒）")) -> ()  [unwired: 1 out]
            }
          }
          frame #5 {
            n13 = property on="进度条" class="Slide (严格)"("Visible"=FALSE ("可见")) -> ()  [unwired: 2 in, 2 out]
          }
        }
        n14 = call <vilib>:"System Exec.vi"("working directory"=path "H:/新", "command line"="matlab -sd H:\\新 -r JJJ1") -> ()  [unwired: 6 in, 4 out]
      }
      event "矩角特性": Value Change {
        n15 = event-data() -> ()  [unwired: 1 in, 6 out]
        n16 = mathscript code="load H:\\新\\J1.mat;\n\n\nplot(ToutJ1(:,2).*1000,WJ1(:,2),'r');\nhold on;\nload H:\\新\\J2.mat;\nplot(ToutJ2(:,2).*1000,WJ2(:,2),'g');\nhold on;\nload H:\\新\\J3.mat;\nplot(ToutJ3(:,2).*1000,WJ3(:,2),'b');\nxlabel('转矩(mNm)');\nylabel('转速(r/min)');\ntitle('矩角特性');\ngrid on;\nlegend('小惯量','中惯量','大惯量');"() -> ()  [unwired: 1 in, 1 out]
      }
      event "输入完成": Value Change {
        w506 = ";"
        w508 = i16 15 ("精度(6)")
        w505 = "\n"
        n17 = event-data() -> ()  [unwired: 1 in, 6 out]
        n18 = Number To Fractional String(number="摩擦材料等效刚度", precision (6)=w508) -> (F-format string=w523:string)  [unwired: 2 in]
        n19 = Number To Fractional String(number="转子等效半径", precision (6)=w508) -> (F-format string=w520:string)  [unwired: 2 in]
        n20 = Number To Fractional String(number="预紧力", precision (6)=w508) -> (F-format string=w514:string)  [unwired: 2 in]
        n21 = Number To Fractional String(number="行波波数", precision (6)=w508) -> (F-format string=w531:string)  [unwired: 2 in]
        n22 = Number To Fractional String(number="转子光电总阻尼", precision (6)=w508) -> (F-format string=w507:string)  [unwired: 2 in]
        n23 = Number To Fractional String(number="定转子间动摩擦系数", precision (6)=w508) -> (F-format string=w526:string)  [unwired: 2 in]
        n24 = Number To Fractional String(number="轴向阻尼系数", precision (6)=w508) -> (F-format string=w517:string)  [unwired: 2 in]
        n25 = Number To Fractional String(number="电机工作频率", precision (6)=w508) -> (F-format string=w511:string)  [unwired: 2 in]
        n26 = Concatenate Strings("%%%%%%%%%总体改变%%%%%%%\n%%%% n 行波波数\n%%%% u 定转子动摩擦系数\n%%%% ke 摩擦材料的等效刚度\n%%%% R 转子等效半径\n%%%% Dz 轴向阻尼系数\n%%%% Dr 转子光电总阻尼\n%%%% Fn 预压力\n%%%%电机工作频率？？？？\n%%%%行波波长？？？？\n%%%%%%%%%%总体改变%%%%%%%%\n%%%%%%%%%%%%%%%%参数值", "\n", "J17=", w531, w506, w505, "J18=", w526, w506, w505, "J19=", w523, w506, w505, "J21=", w520, w506, w505, "J25=", w517, w506, w505, "J26=", w514, w506, w505, "J27=", w511, w506, w505, "J29=", w507, w506, w505, "J30=0.0005;\nJ20=1.5E-03;\nJ22=0.00000066675;\nJ23=0.000000142;\nJ24=0.0005;\nJ28=2*3.1415926*J27;\n\n%%%%%%%%%%%%%%%%%参数值\ngain0=J17/J21;\ngain1=1/gain0;\ngain2=gain0;\ngain3=gain1;\ngain4=2*J18*J19*J22;\ngain5=2;\ngain6=J17*J21;\ngain7=1/J23;\ngain8=J21/gain0/J28;\ngain9=gain1;\ngain10=60/3.1415926/2;\ngain11=2*J17*J19;\ngain12=J25;\ngain13=1/J24;\ngain14=1;\ngain15=gain1;\n%%%%%%%%%%%%%转换为set_para可以用的字符串类型,并且不丢失精度\ntemp=sym(gain0);\ngain0=char(vpa(temp,15));\ntemp=sym(gain1);\ngain1=char(vpa(temp,15));\ntemp=sym(gain2);\ngain2=char(vpa(temp,15));\ntemp=sym(gain3);\ngain3=char(vpa(temp,15));\ntemp=sym(gain4);\ngain4=char(vpa(temp,15));\ntemp=sym(gain5);\ngain5=char(vpa(temp,15));\ntemp=sym(gain6);\ngain6=char(vpa(temp,15));\ntemp=sym(gain7);\ngain7=char(vpa(temp,15));\ntemp=sym(gain8);\ngain8=char(vpa(temp,15));\ntemp=sym(gain9);\ngain9=char(vpa(temp,15));\ntemp=sym(gain10);\ngain10=char(vpa(temp,15));\ntemp=sym(gain11);\ngain11=char(vpa(temp,15));\ntemp=sym(gain12);\ngain12=char(vpa(temp,15));\ntemp=sym(gain13);\ngain13=char(vpa(temp,15));\ntemp=sym(gain14);\ngain14=char(vpa(temp,15));\ntemp=sym(gain15);\ngain15=char(vpa(temp,15));\n%%%将三个simulink模型参数调整\nopen ModerForJ.slx\nset_param('ModerForJ/Gain0','Gain',gain0);\nset_param('ModerForJ/Gain1','Gain',gain1);\nset_param('ModerForJ/Gain2','Gain',gain2);\nset_param('ModerForJ/Gain3','Gain',gain3);\nset_param('ModerForJ/Gain4','Gain',gain4);\nset_param('ModerForJ/Gain5','Gain',gain5);\nset_param('ModerForJ/Gain6','Gain',gain6);\nset_param('ModerForJ/Gain7','Gain',gain7);\nset_param('ModerForJ/Gain8','Gain',gain8);\nset_param('ModerForJ/Gain9','Gain',gain9);\nset_param('ModerForJ/Gain10','Gain',gain10);\nset_param('ModerForJ/Gain11','Gain',gain11);\nset_param('ModerForJ/Gain12','Gain',gain12);\nset_param('ModerForJ/Gain13','Gain',gain13);\nset_param('ModerForJ/Gain14','Gain',gain14);\nset_param('ModerForJ/Gain15','Gain',gain15);\nsave_system;\nclose_system\nopen ModerForT.slx\nset_param('ModerForT/Gain0','Gain',gain0);\nset_param('ModerForT/Gain1','Gain',gain1);\nset_param('ModerForT/Gain2','Gain',gain2);\nset_param('ModerForT/Gain3','Gain',gain3);\nset_param('ModerForT/Gain4','Gain',gain4);\nset_param('ModerForT/Gain5','Gain',gain5);\nset_param('ModerForT/Gain6','Gain',gain6);\nset_param('ModerForT/Gain7','Gain',gain7);\nset_param('ModerForT/Gain8','Gain',gain8);\nset_param('ModerForT/Gain9','Gain',gain9);\nset_param('ModerForT/Gain10','Gain',gain10);\nset_param('ModerForT/Gain11','Gain',gain11);\nset_param('ModerForT/Gain12','Gain',gain12);\nset_param('ModerForT/Gain13','Gain',gain13);\nset_param('ModerForT/Gain14','Gain',gain14);\nset_param('ModerForT/Gain15','Gain',gain15);\nsave_system;\nclose_system\nopen ModerForV.slx\nset_param('ModerForV/Gain0','Gain',gain0);\nset_param('ModerForV/Gain1','Gain',gain1);\nset_param('ModerForV/Gain2','Gain',gain2);\nset_param('ModerForV/Gain3','Gain',gain3);\nset_param('ModerForV/Gain4','Gain',gain4);\nset_param('ModerForV/Gain5','Gain',gain5);\nset_param('ModerForV/Gain6','Gain',gain6);\nset_param('ModerForV/Gain7','Gain',gain7);\nset_param('ModerForV/Gain8','Gain',gain8);\nset_param('ModerForV/Gain9','Gain',gain9);\nset_param('ModerForV/Gain10','Gain',gain10);\nset_param('ModerForV/Gain11','Gain',gain11);\nset_param('ModerForV/Gain12','Gain',gain12);\nset_param('ModerForV/Gain13','Gain',gain13);\nset_param('ModerForV/Gain14','Gain',gain14);\nset_param('ModerForV/Gain15','Gain',gain15);\nsave_system;\nclose_system") -> (w537:string)
        n27 = Open/Create/Replace File(file path (use dialog)=path "H:/新/base.m" ("文件路径（使用对话框）"), operation (0:open)=T2."replace" ("操作(0:open)")) -> (refnum out=w538:refnum<file>)  [unwired: 4 in, 2 out]
        n28 = Write to Text File(file (use dialog)=w538, text=w537) -> (refnum out=w532:refnum<file>)  [unwired: 2 in, 2 out]
        n29 = Close File(refnum=w532) -> ()  [unwired: 1 in, 2 out]
      }
      event "还原按钮": Value Change {
        n30 = event-data() -> ()  [unwired: 1 in, 6 out]
        n31 = Open/Create/Replace File(file path (use dialog)=path "H:/新/base.m" ("文件路径（使用对话框）"), operation (0:open)=T2."replace" ("操作(0:open)")) -> (refnum out=w543:refnum<file>)  [unwired: 4 in, 2 out]
        n32 = Write to Text File(file (use dialog)=w543, text="%%%%%%%%%总体改变%%%%%%%\n%%%% n 行波波数\n%%%% u 定转子动摩擦系数\n%%%% ke 摩擦材料的等效刚度\n%%%% R 转子等效半径\n%%%% Dz 轴向阻尼系数\n%%%% Dr 转子光电总阻尼\n%%%% Fn 预压力\n%%%%电机工作频率？？？？\n%%%%行波波长？？？？\n%%%%%%%%%%总体改变%%%%%%%%\n%%%%%%%%%%%%%%%%参数值\nJ17=9;\nJ18=0.2;\nJ19=2.6E+09;\nJ21=3.10E-03;\nJ25=9300;\nJ26=10;\nJ27=70000;\nJ29=0.00014;\nJ30=0.0005;\nJ20=1.5E-03;\nJ22=0.00000066675;\nJ23=0.000000142;\nJ24=0.0005;\nJ28=2*3.1415926*J27;\n\n%%%%%%%%%%%%%%%%%参数值\ngain0=J17/J21;\ngain1=1/gain0;\ngain2=gain0;\ngain3=gain1;\ngain4=2*J18*J19*J22;\ngain5=2;\ngain6=J17*J21;\ngain7=1/J23;\ngain8=J21/gain0/J28;\ngain9=gain1;\ngain10=60/3.1415926/2;\ngain11=2*J17*J19;\ngain12=J25;\ngain13=1/J24;\ngain14=1;\ngain15=gain1;\n%%%%%%%%%%%%%转换为set_para可以用的字符串类型,并且不丢失精度\ntemp=sym(gain0);\ngain0=char(vpa(temp,15));\ntemp=sym(gain1);\ngain1=char(vpa(temp,15));\ntemp=sym(gain2);\ngain2=char(vpa(temp,15));\ntemp=sym(gain3);\ngain3=char(vpa(temp,15));\ntemp=sym(gain4);\ngain4=char(vpa(temp,15));\ntemp=sym(gain5);\ngain5=char(vpa(temp,15));\ntemp=sym(gain6);\ngain6=char(vpa(temp,15));\ntemp=sym(gain7);\ngain7=char(vpa(temp,15));\ntemp=sym(gain8);\ngain8=char(vpa(temp,15));\ntemp=sym(gain9);\ngain9=char(vpa(temp,15));\ntemp=sym(gain10);\ngain10=char(vpa(temp,15));\ntemp=sym(gain11);\ngain11=char(vpa(temp,15));\ntemp=sym(gain12);\ngain12=char(vpa(temp,15));\ntemp=sym(gain13);\ngain13=char(vpa(temp,15));\ntemp=sym(gain14);\ngain14=char(vpa(temp,15));\ntemp=sym(gain15);\ngain15=char(vpa(temp,15));\n%%%将三个simulink模型参数调整\nopen ModerForJ.slx\nset_param('ModerForJ/Gain0','Gain',gain0);\nset_param('ModerForJ/Gain1','Gain',gain1);\nset_param('ModerForJ/Gain2','Gain',gain2);\nset_param('ModerForJ/Gain3','Gain',gain3);\nset_param('ModerForJ/Gain4','Gain',gain4);\nset_param('ModerForJ/Gain5','Gain',gain5);\nset_param('ModerForJ/Gain6','Gain',gain6);\nset_param('ModerForJ/Gain7','Gain',gain7);\nset_param('ModerForJ/Gain8','Gain',gain8);\nset_param('ModerForJ/Gain9','Gain',gain9);\nset_param('ModerForJ/Gain10','Gain',gain10);\nset_param('ModerForJ/Gain11','Gain',gain11);\nset_param('ModerForJ/Gain12','Gain',gain12);\nset_param('ModerForJ/Gain13','Gain',gain13);\nset_param('ModerForJ/Gain14','Gain',gain14);\nset_param('ModerForJ/Gain15','Gain',gain15);\nsave_system;\nclose_system\nopen ModerForT.slx\nset_param('ModerForT/Gain0','Gain',gain0);\nset_param('ModerForT/Gain1','Gain',gain1);\nset_param('ModerForT/Gain2','Gain',gain2);\nset_param('ModerForT/Gain3','Gain',gain3);\nset_param('ModerForT/Gain4','Gain',gain4);\nset_param('ModerForT/Gain5','Gain',gain5);\nset_param('ModerForT/Gain6','Gain',gain6);\nset_param('ModerForT/Gain7','Gain',gain7);\nset_param('ModerForT/Gain8','Gain',gain8);\nset_param('ModerForT/Gain9','Gain',gain9);\nset_param('ModerForT/Gain10','Gain',gain10);\nset_param('ModerForT/Gain11','Gain',gain11);\nset_param('ModerForT/Gain12','Gain',gain12);\nset_param('ModerForT/Gain13','Gain',gain13);\nset_param('ModerForT/Gain14','Gain',gain14);\nset_param('ModerForT/Gain15','Gain',gain15);\nsave_system;\nclose_system\nopen ModerForV.slx\nset_param('ModerForV/Gain0','Gain',gain0);\nset_param('ModerForV/Gain1','Gain',gain1);\nset_param('ModerForV/Gain2','Gain',gain2);\nset_param('ModerForV/Gain3','Gain',gain3);\nset_param('ModerForV/Gain4','Gain',gain4);\nset_param('ModerForV/Gain5','Gain',gain5);\nset_param('ModerForV/Gain6','Gain',gain6);\nset_param('ModerForV/Gain7','Gain',gain7);\nset_param('ModerForV/Gain8','Gain',gain8);\nset_param('ModerForV/Gain9','Gain',gain9);\nset_param('ModerForV/Gain10','Gain',gain10);\nset_param('ModerForV/Gain11','Gain',gain11);\nset_param('ModerForV/Gain12','Gain',gain12);\nset_param('ModerForV/Gain13','Gain',gain13);\nset_param('ModerForV/Gain14','Gain',gain14);\nset_param('ModerForV/Gain15','Gain',gain15);\nsave_system;\nclose_system" ("文本")) -> (refnum out=w540:refnum<file>)  [unwired: 2 in, 2 out]
        n33 = Close File(refnum=w540) -> ()  [unwired: 1 in, 2 out]
      }
      event "完成": Value Change {
        n34 = event-data() -> ()  [unwired: 1 in, 6 out]
        n35 = Number To Fractional String(number="转动惯量", precision (6)=i16 12 ("精度(6)")) -> (F-format string=w545:string)  [unwired: 2 in]
        n36 = Concatenate Strings("clear;clc;\nopen ModerForJ.slx", "\n", "J=", w545, ";", "\n", "gain7=num2str(1/J);\nset_param('ModerForJ/Gain7','Gain',gain7)\nsim('ModerForJ')\nTJ1=TJ3;\nToutJ1=ToutJ3;\nWJ1=WJ3;\nX0J1=X0J3;\nX1J1=X1J3;\nclear J;\nclear gain7;\nclear TJ3;\nclear tout;\nclear ToutJ3;\nclear WJ3;\nclear X0J3;\nclear X1J3;\nclear yout;\nsave J1.mat\nsave_system;\nexit;") -> (w556:string)
        n37 = Open/Create/Replace File(file path (use dialog)=path "H:/新/JJJ1.m" ("文件路径（使用对话框）"), operation (0:open)=T2."replace" ("操作(0:open)")) -> (refnum out=w557:refnum<file>)  [unwired: 4 in, 2 out]
        n38 = Write to Text File(file (use dialog)=w557, text=w556) -> (refnum out=w547:refnum<file>)  [unwired: 2 in, 2 out]
        n39 = Close File(refnum=w547) -> ()  [unwired: 1 in, 2 out]
      }
      event "完成": Value Change {
        n40 = event-data() -> ()  [unwired: 1 in, 6 out]
        n41 = Number To Fractional String(number="负载转矩1", precision (6)=i16 12 ("精度(6)")) -> (F-format string=w560:string)  [unwired: 2 in]
        n42 = Concatenate Strings("clear;clc;\nopen ModerForT.slx", "\n", "T=", w560, ";", "\n", "T=num2str(T);\nset_param('ModerForT/T','Value',T)\nsim('ModerForT');\nclear T;\nclear tout;\nclear yout;\nsave T1.mat\nsave_system;\nexit;") -> (w570:string)
        n43 = Open/Create/Replace File(file path (use dialog)=path "H:/新/TTT1.m" ("文件路径（使用对话框）"), operation (0:open)=T2."replace" ("操作(0:open)")) -> (refnum out=w571:refnum<file>)  [unwired: 4 in, 2 out]
        n44 = Write to Text File(file (use dialog)=w571, text=w570) -> (refnum out=w561:refnum<file>)  [unwired: 2 in, 2 out]
        n45 = Close File(refnum=w561) -> ()  [unwired: 1 in, 2 out]
      }
      event "完成": Value Change {
        n46 = event-data() -> ()  [unwired: 1 in, 6 out]
        n47 = Number To Fractional String(number="转动惯量", precision (6)=i16 12 ("精度(6)")) -> (F-format string=w572:string)  [unwired: 2 in]
        n48 = Concatenate Strings("clear;clc;\nopen ModerForJ.slx", "\n", "J=", w572, ";", "\n", "gain7=num2str(1/J);\nset_param('ModerForJ/Gain7','Gain',gain7)\nsim('ModerForJ')\nTJ2=TJ3;\nToutJ2=ToutJ3;\nWJ2=WJ3;\nX0J2=X0J3;\nX1J2=X1J3;\nclear J;\nclear gain7;\nclear TJ3;\nclear tout;\nclear ToutJ3;\nclear WJ3;\nclear X0J3;\nclear X1J3;\nclear yout;\nsave J2.mat\nexit") -> (w583:string)
        n49 = Open/Create/Replace File(file path (use dialog)=path "H:/新/JJJ2.m" ("文件路径（使用对话框）"), operation (0:open)=T2."replace" ("操作(0:open)")) -> (refnum out=w584:refnum<file>)  [unwired: 4 in, 2 out]
        n50 = Write to Text File(file (use dialog)=w584, text=w583) -> ()  [unwired: 2 in, 3 out]
      }
      event "完成": Value Change {
        n51 = event-data() -> ()  [unwired: 1 in, 6 out]
        n52 = Number To Fractional String(number="转动惯量", precision (6)=i16 12 ("精度(6)")) -> (F-format string=w585:string)  [unwired: 2 in]
        n53 = Concatenate Strings("clear;clc;\nopen ModerForJ.slx", "\n", "J=", w585, ";", "\n", "gain7=num2str(1/J);\nset_param('ModerForJ/Gain7','Gain',gain7)\nsim('ModerForJ')\n% TJ3=TJ3;\n% ToutJ1=ToutJ3;\n% WJ1=WJ3;\n% X0J1=X0J3;\n% X1J1=X1J3;\nclear J;\nclear gain7;\nclear tout;\nclear yout;\nsave J3.mat\nsave_system;\nexit;") -> (w596:string)
        n54 = Open/Create/Replace File(file path (use dialog)=path "H:/新/JJJ3.m" ("文件路径（使用对话框）"), operation (0:open)=T2."replace" ("操作(0:open)")) -> (refnum out=w597:refnum<file>)  [unwired: 4 in, 2 out]
        n55 = Write to Text File(file (use dialog)=w597, text=w596) -> ()  [unwired: 2 in, 3 out]
      }
      event "完成": Value Change {
        n56 = event-data() -> ()  [unwired: 1 in, 6 out]
        n57 = Number To Fractional String(number="负载转矩2", precision (6)=i16 12 ("精度(6)")) -> (F-format string=w600:string)  [unwired: 2 in]
        n58 = Concatenate Strings("clear;clc;\nopen ModerForT.slx", "\n", "T=", w600, ";", "\n", "T=num2str(T);\nset_param('ModerForT/T','Value',T)\nsim('ModerForT');\nclear T;\nclear tout;\nclear yout;\nToutT2=ToutT1;\nTT2=TT1;\nWT2=WT1;\nsave T2.mat\nsave_system;\nexit;") -> (w610:string)
        n59 = Open/Create/Replace File(file path (use dialog)=path "H:/新/TTT2.m" ("文件路径（使用对话框）"), operation (0:open)=T2."replace" ("操作(0:open)")) -> (refnum out=w611:refnum<file>)  [unwired: 4 in, 2 out]
        n60 = Write to Text File(file (use dialog)=w611, text=w610) -> (refnum out=w601:refnum<file>)  [unwired: 2 in, 2 out]
        n61 = Close File(refnum=w601) -> ()  [unwired: 1 in, 2 out]
      }
      event "完成": Value Change {
        n62 = event-data() -> ()  [unwired: 1 in, 6 out]
        n63 = Number To Fractional String(number="负载转矩3", precision (6)=i16 12 ("精度(6)")) -> (F-format string=w614:string)  [unwired: 2 in]
        n64 = Concatenate Strings("clear;clc;\nopen ModerForT.slx", "\n", "T=", w614, ";", "\n", "T=num2str(T);\nset_param('ModerForT/T','Value',T)\nsim('ModerForT');\nclear T;\nclear tout;\nclear yout;\nToutT3=ToutT1;\nTT3=TT1;\nWT3=WT1;\nsave T3.mat\nsave_system;\nexit;") -> (w624:string)
        n65 = Open/Create/Replace File(file path (use dialog)=path "H:/新/TTT3.m" ("文件路径（使用对话框）"), operation (0:open)=T2."replace" ("操作(0:open)")) -> (refnum out=w625:refnum<file>)  [unwired: 4 in, 2 out]
        n66 = Write to Text File(file (use dialog)=w625, text=w624) -> (refnum out=w615:refnum<file>)  [unwired: 2 in, 2 out]
        n67 = Close File(refnum=w615) -> ()  [unwired: 1 in, 2 out]
      }
      event "完成": Value Change {
        n68 = event-data() -> ()  [unwired: 1 in, 6 out]
        n69 = Number To Fractional String(number="负载转矩4", precision (6)=i16 12 ("精度(6)")) -> (F-format string=w628:string)  [unwired: 2 in]
        n70 = Concatenate Strings("clear;clc;\nopen ModerForT.slx", "\n", "T=", w628, ";", "\n", "T=num2str(T);\nset_param('ModerForT/T','Value',T)\nsim('ModerForT');\nclear T;\nclear tout;\nclear yout;\nToutT4=ToutT1;\nTT4=TT1;\nWT4=WT1;\nsave T4.mat\nsave_system;\nexit;") -> (w638:string)
        n71 = Open/Create/Replace File(file path (use dialog)=path "H:/新/TTT4.m" ("文件路径（使用对话框）"), operation (0:open)=T2."replace" ("操作(0:open)")) -> (refnum out=w639:refnum<file>)  [unwired: 4 in, 2 out]
        n72 = Write to Text File(file (use dialog)=w639, text=w638) -> (refnum out=w629:refnum<file>)  [unwired: 2 in, 2 out]
        n73 = Close File(refnum=w629) -> ()  [unwired: 1 in, 2 out]
      }
      event "启动特性": Value Change {
        n74 = event-data() -> ()  [unwired: 1 in, 6 out]
        n75 = mathscript code="load H:\\新\\J1.mat;\n\n\nplot(WJ1(:,1).*1000,WJ1(:,2),'r');\nhold on;\nload H:\\新\\J2.mat;\nplot(WJ2(:,1).*1000,WJ2(:,2),'g');\nhold on;\nload H:\\新\\J3.mat;\nplot(WJ3(:,1).*1000,WJ3(:,2),'b');\nxlabel('时间(ms)');\nylabel('转速(r/min)');\ntitle('启动特性');\ngrid on;\nlegend('小惯量','中惯量','大惯量');"() -> ()  [unwired: 1 in, 1 out]
      }
      event Value Change {
        n76 = event-data() -> ()  [unwired: 1 in, 6 out]
        n77 = call <vilib>:"System Exec.vi"("working directory"=path "H:/新", "command line"="matlab -sd H:\\新 -r JJJ2") -> ()  [unwired: 6 in, 4 out]
      }
      event Value Change {
        n78 = event-data() -> ()  [unwired: 1 in, 6 out]
        n79 = call <vilib>:"System Exec.vi"("working directory"=path "H:/新", "command line"="matlab -sd H:\\新 -r VVV1") -> ()  [unwired: 6 in, 4 out]
      }
      event Value Change {
        n80 = event-data() -> ()  [unwired: 1 in, 6 out]
        n81 = call <vilib>:"System Exec.vi"("working directory"=path "H:/新", "command line"="matlab -sd H:\\新 -r VVV2") -> ()  [unwired: 6 in, 4 out]
      }
      event Value Change {
        n82 = event-data() -> ()  [unwired: 1 in, 6 out]
        n83 = call <vilib>:"System Exec.vi"("working directory"=path "H:/新", "command line"="matlab -sd H:\\新 -r VVV3") -> ()  [unwired: 6 in, 4 out]
      }
      event "启动特性": Value Change {
        n84 = event-data() -> ()  [unwired: 1 in, 6 out]
        n85 = mathscript code="load H:\\新\\V1.mat;\n\nplot(WV1(:,1).*1000,WV1(:,2),'r');\nhold on;\nload H:\\新\\V2.mat;\n\nplot(WV2(:,1).*1000,WV2(:,2),'g');\nhold on;\nload H:\\新\\V3.mat;\nplot(WV3(:,1).*1000,WV3(:,2),'b');\nxlabel('时间(ms)');\nylabel('转速(r/min)');\ntitle('启动特性');\ngrid on;\nlegend('小振幅','中振幅','大振幅');"() -> ()  [unwired: 1 in, 1 out]
      }
      event "摩擦转矩-转速": Value Change {
        n86 = event-data() -> ()  [unwired: 1 in, 6 out]
        n87 = mathscript code="load H:\\新\\V1.mat;\n\nplot(TV1(:,2).*1000,WV1(:,2),'r');\nhold on;\nload H:\\新\\V2.mat;\n\nplot(TV2(:,2).*1000,WV2(:,2),'g');\nhold on;\nload H:\\新\\V3.mat;\nplot(TV3(:,2).*1000,WV3(:,2),'b');\nxlabel('转矩(mNm)');\nylabel('转速(r/min)');\ntitle('总摩擦转矩-转速特性');\ngrid on;\nlegend('小振幅','中振幅','大振幅');"() -> ()  [unwired: 1 in, 1 out]
      }
      event "矩角特性": Value Change {
        n88 = event-data() -> ()  [unwired: 1 in, 6 out]
        n89 = mathscript code="load H:\\新\\V1.mat;\n\nplot(ToutV1(:,2).*1000,WV1(:,2),'r');\nhold on;\nload H:\\新\\V2.mat;\n\nplot(ToutV2(:,2).*1000,WV2(:,2),'g');\nhold on;\nload H:\\新\\V3.mat;\nplot(ToutV3(:,2).*1000,WV3(:,2),'b');\nxlabel('转矩(mNm)');\nylabel('转速(r/min)');\ntitle('矩角特性');\ngrid on;\nlegend('小振幅','中振幅','大振幅');"() -> ()  [unwired: 1 in, 1 out]
      }
      event Value Change {
        n90 = event-data() -> ()  [unwired: 1 in, 6 out]
        n91 = call <vilib>:"System Exec.vi"("working directory"=path "H:/新", "command line"="matlab -sd H:\\新 -r TTT1") -> ()  [unwired: 6 in, 4 out]
      }
      event "完成": Value Change {
        n92 = event-data() -> ()  [unwired: 1 in, 6 out]
        n93 = Number To Fractional String(number="定子形波振幅", precision (6)=i16 12 ("精度(6)")) -> (F-format string=w2611:string)  [unwired: 2 in]
        n94 = Concatenate Strings("clear;clc;\nopen ModerForV.slx", "\n", "V=", w2611, ";", "\n", "V=num2str(V);\nset_param('ModerForV/V','Value',V);\nclear V;\nsim('ModerForV');\nclear tout;\nclear yout;\nsave V1.mat\nsave_system;\nexit;") -> (w2621:string)
        n95 = Open/Create/Replace File(file path (use dialog)=path "H:/新/VVV1.m" ("文件路径（使用对话框）"), operation (0:open)=T2."replace" ("操作(0:open)")) -> (refnum out=w2622:refnum<file>)  [unwired: 4 in, 2 out]
        n96 = Write to Text File(file (use dialog)=w2622, text=w2621) -> ()  [unwired: 2 in, 3 out]
      }
      event "完成": Value Change {
        n97 = event-data() -> ()  [unwired: 1 in, 6 out]
        n98 = Number To Fractional String(number="定子形波振幅2", precision (6)=i16 12 ("精度(6)")) -> (F-format string=w2624:string)  [unwired: 2 in]
        n99 = Concatenate Strings("clear;clc;\nopen ModerForV.slx", "\n", "V=", w2624, ";", "\n", "V=num2str(V);\nset_param('ModerForV/V','Value',V);\nclear V;\nsim('ModerForV');\nclear tout;\nclear yout;\nFZV2=FZV1;\nToutV2=ToutV1;\nTV2=TV1;\nWV2=WV1;\nX0V2=X0V1;\nX1V2=X1V1;\nsave V2.mat\nsave_system;\nexit;") -> (w2634:string)
        n100 = Open/Create/Replace File(file path (use dialog)=path "H:/新/VVV2.m" ("文件路径（使用对话框）"), operation (0:open)=T2."replace" ("操作(0:open)")) -> (refnum out=w2635:refnum<file>)  [unwired: 4 in, 2 out]
        n101 = Write to Text File(file (use dialog)=w2635, text=w2634) -> ()  [unwired: 2 in, 3 out]
      }
      event "完成": Value Change {
        n102 = event-data() -> ()  [unwired: 1 in, 6 out]
        n103 = Number To Fractional String(number="定子形波振幅3", precision (6)=i16 12 ("精度(6)")) -> (F-format string=w2637:string)  [unwired: 2 in]
        n104 = Concatenate Strings("clear;clc;\nopen ModerForV.slx", "\n", "V=", w2637, ";", "\n", "V=num2str(V);\nset_param('ModerForV/V','Value',V);\nclear V;\nsim('ModerForV');\nclear tout;\nclear yout;\nFZV3=FZV1;\nToutV3=ToutV1;\nTV3=TV1;\nWV3=WV1;\nX0V3=X0V1;\nX1V3=X1V1;\nsave V3.mat\nsave_system;\nexit;") -> (w2647:string)
        n105 = Open/Create/Replace File(file path (use dialog)=path "H:/新/VVV2.m" ("文件路径（使用对话框）"), operation (0:open)=T2."replace" ("操作(0:open)")) -> (refnum out=w2648:refnum<file>)  [unwired: 4 in, 2 out]
        n106 = Write to Text File(file (use dialog)=w2648, text=w2647) -> ()  [unwired: 2 in, 3 out]
      }
      event Value Change {
        n107 = event-data() -> ()  [unwired: 1 in, 6 out]
        n108 = call <vilib>:"System Exec.vi"("working directory"=path "H:/新", "command line"="matlab -sd H:\\新 -r TTT2") -> ()  [unwired: 6 in, 4 out]
      }
      event Value Change {
        n109 = event-data() -> ()  [unwired: 1 in, 6 out]
        n110 = call <vilib>:"System Exec.vi"("working directory"=path "H:/新", "command line"="matlab -sd H:\\新 -r TTT3") -> ()  [unwired: 6 in, 4 out]
      }
      event "净输出转矩-转速关系": Value Change {
        n111 = event-data() -> ()  [unwired: 1 in, 6 out]
        n112 = mathscript code="load H:\\新\\T1.mat;\nplot(ToutT1(:,2).*1000,WT1(:,2),'r');\nhold on;\nload H:\\新\\T2.mat;\nplot(ToutT2(:,2).*1000,WT2(:,2),'g');\nhold on;\nload H:\\新\\T3.mat;\nplot(ToutT3(:,2).*1000,WT3(:,2),'b');\nhold on;\nload H:\\新\\T4.mat;\nplot(ToutT4(:,2).*1000,WT4(:,2),'p');\nxlabel('转矩(mNm)');\nylabel('转速(r/min)');\ntitle('负载转矩-转速特性');\ngrid on;\nlegend(' 0 mNm负载',' 5 mNm负载',' 8 mNm负载','10mNm负载');"() -> ()  [unwired: 1 in, 1 out]
      }
      event "矩角特性": Value Change {
        n113 = event-data() -> ()  [unwired: 1 in, 6 out]
        n114 = mathscript code="load H:\\新\\T1.mat;\nplot(ToutT1(:,2).*1000,WT1(:,2),'r');\nhold on;\nload H:\\新\\T2.mat;\nplot(ToutT2(:,2).*1000+5.0,WT2(:,2),'g');\nhold on;\nload H:\\新\\T3.mat;\nplot(ToutT3(:,2).*1000+8.0,WT3(:,2),'b');\nhold on;\nload H:\\新\\T4.mat;\nplot(TT4(:,2).*1000-5.0,WT4(:,2),'p');\nxlabel('转矩(mNm)');\nylabel('转速(r/min)');\ntitle('矩角特性');\ngrid on;\nlegend(' 0 mNm负载',' 5 mNm负载',' 8 mNm负载','10mNm负载');"() -> ()  [unwired: 1 in, 1 out]
      }
      event "启动特性": Value Change {
        n115 = event-data() -> ()  [unwired: 1 in, 6 out]
        n116 = mathscript code="load H:\\新\\T1.mat;\nplot(WT1(:,1).*1000,WT1(:,2),'r');\nhold on;\nload H:\\新\\T2.mat;\nplot(WT2(:,1).*1000,WT2(:,2),'g');\nhold on;\nload H:\\新\\T3.mat;\nplot(WT3(:,1).*1000,WT3(:,2),'b');\nhold on;\nload H:\\新\\T4.mat;\nplot(WT4(:,1).*1000,WT4(:,2),'p');\nxlabel('时间(ms)');\nylabel('转速(r/min)');\ntitle('启动特性');\ngrid on;\nlegend(' 0 mNm负载',' 5 mNm负载',' 8 mNm负载','10mNm负载');"() -> ()  [unwired: 1 in, 1 out]
      }
      event Value Change {
        n117 = event-data() -> ()  [unwired: 1 in, 6 out]
        n118 = call <vilib>:"System Exec.vi"("working directory"=path "H:/新", "command line"="matlab -sd H:\\新 -r TTT4") -> ()  [unwired: 6 in, 4 out]
      }
      event Value Change {
        n119 = event-data() -> ()  [unwired: 1 in, 6 out]
        n120 = call <vilib>:"System Exec.vi"("working directory"=path "H:/新", "command line"="matlab -sd H:\\新 -r JJJ3") -> ()  [unwired: 6 in, 4 out]
      }
    }
  }
  n121 = property on="进度条" class="Slide (严格)"("Visible"=FALSE ("可见")) -> ()  [unwired: 2 in, 2 out]
